vi "20200213_CHF_336.vi"() -> ()   [LabVIEW 2017]
uses:
  <vilib>/DAQmx/miscellaneous.llb/DAQmx Fill In Error Info.vi
  <vilib>/DAQmx/create/channels.llb/DAQmx Create Channel (AI-Voltage-Basic).vi
  <vilib>/DAQmx/create/channels.llb/DAQmx Create Channel (AO-Voltage-Basic).vi
  istr.lib/Lake Shore 336/Public/Data/Sensor Data (Single Reading).vi
  istr.lib/Lake Shore Cryotronics 218.lvlib
  istr.lib/Lake Shore 336/Lake Shore 336.lvlib
panel:
  in  "Tab Control":T1(tab)=enum."graphs"
  out "error out\n(file creation)":errorcluster
  out "error out\n(DAQ config)":errorcluster
  out "error out (LSI)":errorcluster
  out "error out (decoration)":errorcluster
  out "error out (DAQ AOU)":errorcluster
  out "error out (DAQ AIN)":errorcluster
  out "DAQ AIN task out":refnum<k21>="20200318_131117_AI"
  out "error out (end)":errorcluster
  in  "comments LSIU (not recorded)":string[](array[string])=["PtCo", "", "", "", "CERNOX", "CERNOX", "CERNOX", "CERNOX"]
  in  "LSI-U CH labels":string[](array[string])=["NC", "NC", "NC", "NC", "NC", "NC", "NC", "NC"]
  in  "DAQ-AIN labels":string[](array[string])=["P_4KRES", "LM_110", "DP_3He", "DP_4He", "FM_4He", "FM_3He", "LM_1700", "P_3He_IN", "P_3He_OUT", "P_bar_front", "Heater_V", "Heater_I", "LD_exponent", "LD_mantissa", "LD_full"]
  in  "DAQ AIN channels":tag[](array[tag])=["Dev1/ai1", "Dev1/ai2", "Dev1/ai3", "Dev1/ai4", "Dev1/ai5", "Dev1/ai6", "Dev1/ai7", "Dev1/ai16", "Dev1/ai17", "Dev1/ai18", "Dev1/ai19", "Dev1/ai23", "Dev1/ai21", "Dev1/ai22"]
  in  "V_min(in)":dbl[](array[numeric])=[0.0, 0.0, 0.0, 0.0, 0.0, 0.0, 0.0, 0.0, 0.0, 0.0, 0.0, 0.0, 0.0, 0.0]
  in  "V_max(in)":dbl[](array[numeric])=[5.0, 0.15, 5.0, 5.0, 5.0, 5.0, 10.0, 5.0, 5.0, 5.0, 10.0, 10.0, 10.0, 10.0]
  in  "comments DAQ (not recorded)":string[](array[string])=["", "", "pressure diff., range : 0-20kPa", "pressure diff., rrange : 0-1kPa", "", "", "The range of this is 0-10VDC", "absoulte pressure, 1-5V <-> 0-200kPa", "absoulte pressure, 1-5V <-> 0-200kPa", "baratron analog out ", "voltage over the heater via a voltage divider ", "current in A which flows through the heater", "leak detector readou exponent ", "leak detector readout mantissa"]
  in  "DAQ sample #":i32=5
  in  "LSI-D CH labels":string[](array[string])=["Helium", "Cu", "NC", "NC", "NC", "NC", "NC", "NC"]
  in  "comments LSID (not recorded)":string[](array[string])=["", "", "PtCo", "PtCo", "CERNOX", "CERNOX", "CERNOX", "CERNOX"]
  in  "VISA LSI218 UP":refnum<visa-resource-name>="GPIB0::8::INSTR"
  in  "VISA LSI336":refnum<visa-resource-name>="GPIB0::1::INSTR"
  in  "Rv/(Rv+Ro)":dbl=0.0907441 format="%_7f"
  in  "Ri (Ohm)":dbl=10.1 format="%_4f"
  out "DAQ AIN CONV":dbl[](array[numeric])=[-48461.36222166339, -0.034257721777445925, 46.07595449774182, 23.305171113781608, 0.6935562473065429, 0.15116757050047003, 0.036201034541511884, 100765.895313031, 101089.75178250414, 99597.26569585872, 0.010176692246159401, -5.8343379889446384e-05, -2.0, -0.004535554012344961, -4.535554012344961e-05]
  out "DAQ RAW":dbl[](array[numeric])=[0.04675189478348817, -0.00015003007966136236, 1.0071438225092348, 1.102328129093408, 0.014037402194859598, -0.0002649139326618283, 0.0025019891266333943, 3.0153836639221887, 3.0379056620474696, 3.940429396233107, -0.0017731538983390277, -0.00012886811862497516, 0.009407989382065898, -0.0011154395863216121, 0.0]
  out "LSI-D CH indic.":string[](array[string])=["Helium", "Cu", "NC", "NC", "NC", "NC", "NC", "NC"]
  out "LSI-D out":dbl[](array[numeric])=[0.0, 0.0, 1.213, 0.0, 0.0, 0.0, 4.0, 4.0]
  out "LSI-U CH indic,":string[](array[string])=["NC", "NC", "NC", "NC", "NC", "NC", "NC", "NC"]
  out "LSI-U out":dbl[](array[numeric])=[286.694, 286.481, 0.0, 0.0, 0.0, 0.0, 0.0, 0.0]
  out "DAQ AIN CH indic.":string[](array[string])=["P_4KRES", "LM_110", "DP_3He", "DP_4He", "FM_4He", "FM_3He", "LM_1700", "P_3He_IN", "P_3He_OUT", "P_bar_front", "Heater_V", "Heater_I", "LD_exponent", "LD_mantissa", "LD_full"]
  in  "log/linear 4":bool
  out "Graph LSI-D 1":cluster{dbl[], dbl[]}[](graph)=[{[3667349478.0127354, 3667349479.0140834, 3667349480.0134497, 3667349481.013572, 3667349482.014925, 3667349483.014216, 3667349484.015578, 3667349485.016135, 3667349486.016583, 3667349487.0163903, 3667349488.0179815, 3667349489.018835, 3667349490.018664, 3667349491.0187654, 3667349492.0187993, 3667349493.019667, 3667349494.019672, 3667349495.0196695, 3667349496.019436, 3667349497.021096, 3667349498.0206184], [0.0, 0.0, 0.0, 0.0, 0.0, 0.0, 0.0, 0.0, 0.0, 0.0, 0.0, 0.0, 0.0, 0.0, 0.0, 0.0, 0.0, 0.0, 0.0, 0.0, 0.0]}, {[3667349478.0127354, 3667349479.0140834, 3667349480.0134497, 3667349481.013572, 3667349482.014925, 3667349483.014216, 3667349484.015578, 3667349485.016135, 3667349486.016583, 3667349487.0163903, 3667349488.0179815, 3667349489.018835, 3667349490.018664, 3667349491.0187654, 3667349492.0187993, 3667349493.019667, 3667349494.019672, 3667349495.0196695, 3667349496.019436, 3667349497.021096, 3667349498.0206184], [0.0, 0.0, 0.0, 0.0, 0.0, 0.0, 0.0, 0.0, 0.0, 0.0, 0.0, 0.0, 0.0, 0.0, 0.0, 0.0, 0.0, 0.0, 0.0, 0.0, 0.0]}, {[3667349478.0127354, 3667349479.0140834, 3667349480.0134497, 3667349481.013572, 3667349482.014925, 3667349483.014216, 3667349484.015578, 3667349485.016135, 3667349486.016583, 3667349487.0163903, 3667349488.0179815, 3667349489.018835, 3667349490.018664, 3667349491.0187654, 3667349492.0187993, 3667349493.019667, 3667349494.019672, 3667349495.0196695, 3667349496.019436, 3667349497.021096, 3667349498.0206184], [1.213, 1.213, 1.213, 1.213, 1.213, 1.213, 1.213, 1.213, 1.213, 1.213, 1.213, 1.213, 1.213, 1.213, 1.213, 1.213, 1.213, 1.213, 1.213, 1.213, 1.213]}, {[3667349478.0127354, 3667349479.0140834, 3667349480.0134497, 3667349481.013572, 3667349482.014925, 3667349483.014216, 3667349484.015578, 3667349485.016135, 3667349486.016583, 3667349487.0163903, 3667349488.0179815, 3667349489.018835, 3667349490.018664, 3667349491.0187654, 3667349492.0187993, 3667349493.019667, 3667349494.019672, 3667349495.0196695, 3667349496.019436, 3667349497.021096, 3667349498.0206184], [0.0, 0.0, 0.0, 0.0, 0.0, 0.0, 0.0, 0.0, 0.0, 0.0, 0.0, 0.0, 0.0, 0.0, 0.0, 0.0, 0.0, 0.0, 0.0, 0.0, 0.0]}, {[3667349478.0127354, 3667349479.0140834, 3667349480.0134497, 3667349481.013572, 3667349482.014925, 3667349483.014216, 3667349484.015578, 3667349485.016135, 3667349486.016583, 3667349487.0163903, 3667349488.0179815, 3667349489.018835, 3667349490.018664, 3667349491.0187654, 3667349492.0187993, 3667349493.019667, 3667349494.019672, 3667349495.0196695, 3667349496.019436, 3667349497.021096, 3667349498.0206184], [0.0, 0.0, 0.0, 0.0, 0.0, 0.0, 0.0, 0.0, 0.0, 0.0, 0.0, 0.0, 0.0, 0.0, 0.0, 0.0, 0.0, 0.0, 0.0, 0.0, 0.0]}, {[3667349478.0127354, 3667349479.0140834, 3667349480.0134497, 3667349481.013572, 3667349482.014925, 3667349483.014216, 3667349484.015578, 3667349485.016135, 3667349486.016583, 3667349487.0163903, 3667349488.0179815, 3667349489.018835, 3667349490.018664, 3667349491.0187654, 3667349492.0187993, 3667349493.019667, 3667349494.019672, 3667349495.0196695, 3667349496.019436, 3667349497.021096, 3667349498.0206184], [0.0, 0.0, 0.0, 0.0, 0.0, 0.0, 0.0, 0.0, 0.0, 0.0, 0.0, 0.0, 0.0, 0.0, 0.0, 0.0, 0.0, 0.0, 0.0, 0.0, 0.0]}, {[3667349478.0127354, 3667349479.0140834, 3667349480.0134497, 3667349481.013572, 3667349482.014925, 3667349483.014216, 3667349484.015578, 3667349485.016135, 3667349486.016583, 3667349487.0163903, 3667349488.0179815, 3667349489.018835, 3667349490.018664, 3667349491.0187654, 3667349492.0187993, 3667349493.019667, 3667349494.019672, 3667349495.0196695, 3667349496.019436, 3667349497.021096, 3667349498.0206184], [4.0, 4.0, 4.0, 4.0, 4.0, 4.0, 4.0, 4.0, 4.0, 4.0, 4.0, 4.0, 4.0, 4.0, 4.0, 4.0, 4.0, 4.0, 4.0, 4.0, 4.0]}, {[3667349478.0127354, 3667349479.0140834, 3667349480.0134497, 3667349481.013572, 3667349482.014925, 3667349483.014216, 3667349484.015578, 3667349485.016135, 3667349486.016583, 3667349487.0163903, 3667349488.0179815, 3667349489.018835, 3667349490.018664, 3667349491.0187654, 3667349492.0187993, 3667349493.019667, 3667349494.019672, 3667349495.0196695, 3667349496.019436, 3667349497.021096, 3667349498.0206184], [4.0, 4.0, 4.0, 4.0, 4.0, 4.0, 4.0, 4.0, 4.0, 4.0, 4.0, 4.0, 4.0, 4.0, 4.0, 4.0, 4.0, 4.0, 4.0, 4.0, 4.0]}, {[3667349478.0127354, 3667349479.0140834, 3667349480.0134497, 3667349481.013572, 3667349482.014925, 3667349483.014216, 3667349484.015578, 3667349485.016135, 3667349486.016583, 3667349487.0163903, 3667349488.0179815, 3667349489.018835, 3667349490.018664, 3667349491.0187654, 3667349492.0187993, 3667349493.019667, 3667349494.019672, 3667349495.0196695, 3667349496.019436, 3667349497.021096, 3667349498.0206184], []}] caption="XY Graph"
  out "LSI-D out 1":dbl[](array[numeric])=[0.0, 0.0, 1.213, 0.0, 0.0, 0.0, 4.0, 4.0] format="%_3f"
  in  "log/linear 3":bool
  out "Graph S.1.3":cluster{dbl[], dbl[]}[](graph)=[{[3667349478.0127354, 3667349479.0140834, 3667349480.0134497, 3667349481.013572, 3667349482.014925, 3667349483.014216, 3667349484.015578, 3667349485.016135, 3667349486.016583, 3667349487.0163903, 3667349488.0179815, 3667349489.018835, 3667349490.018664, 3667349491.0187654, 3667349492.0187993, 3667349493.019667, 3667349494.019672, 3667349495.0196695, 3667349496.019436, 3667349497.021096, 3667349498.0206184], [-50521.2245456328, -51001.2563087499, -51385.9392869464, -50463.68651918715, -49646.64610974649, -49625.27485044931, -49894.88173933904, -50284.49655313725, -50743.15703962915, -50720.14180188283, -50039.54881966669, -49418.13787551146, -50679.04319398615, -49158.394647200206, -51098.24902658315, -50233.53425326837, -49625.27484957506, -50683.97503597823, -49748.570680075805, -49692.67657635927, -48461.36222166339]}, {[3667349478.0127354, 3667349479.0140834, 3667349480.0134497, 3667349481.013572, 3667349482.014925, 3667349483.014216, 3667349484.015578, 3667349485.016135, 3667349486.016583, 3667349487.0163903, 3667349488.0179815, 3667349489.018835, 3667349490.018664, 3667349491.0187654, 3667349492.0187993, 3667349493.019667, 3667349494.019672, 3667349495.0196695, 3667349496.019436, 3667349497.021096, 3667349498.0206184], [0.019681672163247236, -0.035573316743868315, -0.023732961916967353, -0.014523797115791916, -0.04609807649843742, 0.003894532544932317, -0.005314632339753402, -0.08425033110491678, -0.08161914105921124, -0.15660805460255026, -0.12898056031693128, -0.04215129156293204, -0.09609068567214586, -0.06714759614249097, 0.04073119171338225, -0.0026834424424830236, -0.13161175006152215, -0.07504116619060815, -0.05004486144342974, -0.043466886677967234, -0.034257721777445925]}, {[3667349478.0127354, 3667349479.0140834, 3667349480.0134497, 3667349481.013572, 3667349482.014925, 3667349483.014216, 3667349484.015578, 3667349485.016135, 3667349486.016583, 3667349487.0163903, 3667349488.0179815, 3667349489.018835, 3667349490.018664, 3667349491.0187654, 3667349492.0187993, 3667349493.019667, 3667349494.019672, 3667349495.0196695, 3667349496.019436, 3667349497.021096, 3667349498.0206184], [38.84260441471943, 39.006998855943834, 54.295670261381716, 29.965311373603143, 57.41916227904098, 16.649371673914672, 23.2251443857745, 16.978160296654554, 20.923623945936498, 25.855453443481835, 63.17296338630207, 33.74638070680503, 32.43122613515559, 37.363055655882384, 31.773648868628214, 29.965311397649465, 28.321368183241713, 23.882721679537866, 22.403172749733137, 59.22749982166353, 46.07595449774182]}, {[3667349478.0127354, 3667349479.0140834, 3667349480.0134497, 3667349481.013572, 3667349482.014925, 3667349483.014216, 3667349484.015578, 3667349485.016135, 3667349486.016583, 3667349487.0163903, 3667349488.0179815, 3667349489.018835, 3667349490.018664, 3667349491.0187654, 3667349492.0187993, 3667349493.019667, 3667349494.019672, 3667349495.0196695, 3667349496.019436, 3667349497.021096, 3667349498.0206184], [23.37092883661357, 22.721571321651922, 21.480394293207027, 24.02028635389264, 23.420247124279147, 23.08323879869223, 23.420247130213735, 22.713351606428176, 21.439295716348617, 23.214754246681622, 22.713351601179323, 23.206534532026367, 21.521492871998007, 22.828427616938708, 23.855892046718395, 22.129751813377673, 23.658618875732728, 22.302365835317307, 21.83384205492711, 21.54615201050991, 23.305171113781608]}, {[3667349478.0127354, 3667349479.0140834, 3667349480.0134497, 3667349481.013572, 3667349482.014925, 3667349483.014216, 3667349484.015578, 3667349485.016135, 3667349486.016583, 3667349487.0163903, 3667349488.0179815, 3667349489.018835, 3667349490.018664, 3667349491.0187654, 3667349492.0187993, 3667349493.019667, 3667349494.019672, 3667349495.0196695, 3667349496.019436, 3667349497.021096, 3667349498.0206184], [0.23982759672010165, 0.26941859522093714, 0.07872104719398296, 0.32531270582554006, -0.01662772910205959, -0.026491393526181937, 0.1806455987303783, 0.4897071440762254, -0.13170383494884252, 0.9565873491766973, 0.17078193234429023, 0.700132025147448, 0.6705410269020168, 0.627798472326523, 0.17406982087029635, 0.476555589056135, 0.48641925466059627, 0.0524179352505974, 0.21023659743522313, 0.06885738001278591, 0.6935562473065429]}, {[3667349478.0127354, 3667349479.0140834, 3667349480.0134497, 3667349481.013572, 3667349482.014925, 3667349483.014216, 3667349484.015578, 3667349485.016135, 3667349486.016583, 3667349487.0163903, 3667349488.0179815, 3667349489.018835, 3667349490.018664, 3667349491.0187654, 3667349492.0187993, 3667349493.019667, 3667349494.019672, 3667349495.0196695, 3667349496.019436, 3667349497.021096, 3667349498.0206184], [-0.0566270005152093, 0.19193739136287796, 0.1327553934585839, 0.15116757047502127, 0.14985241484089812, 0.028858107945263556, -0.040845134196314414, 0.09198557214999697, 0.09856134994531957, -0.08293011069980677, 0.11828868263099351, 0.009130775162069726, 0.07225823943248261, 0.09067041687947358, 0.06962792881441743, 0.10119166098595678, 0.11434321594263724, 0.047270285163107995, 0.024912641362354437, 0.18273130267201193, 0.15116757050047003]}, {[3667349478.0127354, 3667349479.0140834, 3667349480.0134497, 3667349481.013572, 3667349482.014925, 3667349483.014216, 3667349484.015578, 3667349485.016135, 3667349486.016583, 3667349487.0163903, 3667349488.0179815, 3667349489.018835, 3667349490.018664, 3667349491.0187654, 3667349492.0187993, 3667349493.019667, 3667349494.019672, 3667349495.0196695, 3667349496.019436, 3667349497.021096, 3667349498.0206184], [-0.920115595447706, -0.20123383292462396, -0.08218754169592701, 0.01712731949638921, 0.03488560589534542, 0.02304674833120446, 0.023046748329272143, 0.05132846367878108, 0.06514046419026112, 0.0217313197057645, 0.051328463673510655, 0.026335319880004177, 0.047382177823100224, 0.046724463511654324, 0.012523319345340012, -0.0045772527613157366, 0.011207890716825375, 0.015811890907051346, 0.04738217781528495, 0.055932463852581854, 0.036201034541511884]}, {[3667349478.0127354, 3667349479.0140834, 3667349480.0134497, 3667349481.013572, 3667349482.014925, 3667349483.014216, 3667349484.015578, 3667349485.016135, 3667349486.016583, 3667349487.0163903, 3667349488.0179815, 3667349489.018835, 3667349490.018664, 3667349491.0187654, 3667349492.0187993, 3667349493.019667, 3667349494.019672, 3667349495.0196695, 3667349496.019436, 3667349497.021096, 3667349498.0206184], [101084.81995907212, 100790.55443522778, 100880.97121607444, 100578.48598462425, 100890.83486492698, 100798.77414238652, 100728.08465890236, 100733.01648361162, 100821.78932327892, 100805.34990845669, 100811.92567437782, 100746.16801531675, 100894.1227478334, 100876.03939176453, 100568.62233567455, 100836.58479647475, 100622.87240454755, 100854.66815272612, 100912.20610427913, 100640.95576074878, 100765.895313031]}, {[3667349478.0127354, 3667349479.0140834, 3667349480.0134497, 3667349481.013572, 3667349482.014925, 3667349483.014216, 3667349484.015578, 3667349485.016135, 3667349486.016583, 3667349487.0163903, 3667349488.0179815, 3667349489.018835, 3667349490.018664, 3667349491.0187654, 3667349492.0187993, 3667349493.019667, 3667349494.019672, 3667349495.0196695, 3667349496.019436, 3667349497.021096, 3667349498.0206184], [101867.33609569666, 101987.34382303612, 100686.98611819187, 100535.74350397852, 101033.85777256651, 101078.24418841764, 101168.66097001858, 100936.86522534626, 101331.41117828828, 101622.3888165227, 101430.04766636596, 101250.85804619722, 101135.78214419658, 101701.29800932095, 101314.97176400454, 100908.91821834628, 100788.91049122188, 101416.8961349039, 101628.96458413133, 101282.0929351607, 101089.75178250414]}, {[3667349478.0127354, 3667349479.0140834, 3667349480.0134497, 3667349481.013572, 3667349482.014925, 3667349483.014216, 3667349484.015578, 3667349485.016135, 3667349486.016583, 3667349487.0163903, 3667349488.0179815, 3667349489.018835, 3667349490.018664, 3667349491.0187654, 3667349492.0187993, 3667349493.019667, 3667349494.019672, 3667349495.0196695, 3667349496.019436, 3667349497.021096, 3667349498.0206184], [101420.21419989626, 98144.87117860923, 98203.7358752945, 101313.85089177152, 101040.85716494694, 101526.68917410531, 101253.1219474301, 101465.83265061265, 100572.4245095208, 100965.15620313674, 101496.25635307128, 99254.47902652802, 101374.61625787482, 99209.8547871812, 101359.42150088456, 99746.67239306087, 99552.48733932934, 100316.46473552707, 100542.27772973066, 100889.51195743452, 99597.26569585872]}, {[3667349478.0127354, 3667349479.0140834, 3667349480.0134497, 3667349481.013572, 3667349482.014925, 3667349483.014216, 3667349484.015578, 3667349485.016135, 3667349486.016583, 3667349487.0163903, 3667349488.0179815, 3667349489.018835, 3667349490.018664, 3667349491.0187654, 3667349492.0187993, 3667349493.019667, 3667349494.019672, 3667349495.0196695, 3667349496.019436, 3667349497.021096, 3667349498.0206184], [0.018149505272345223, 0.0072774875169589, 0.00582788514456583, -0.00794333736102738, -0.010117740914873347, 0.018874306457283163, 0.006552686320306795, -0.00721853618344779, 0.019599107644447382, 0.00945189105599304, 0.015250300537917006, -0.002144927894012446, 0.009451891063447862, -0.020989758718289512, -0.012292144465621163, 0.0014790780319362934, 0.020323908801802685, -0.026788168204768564, 0.0007542768560017767, 0.0029286803972630835, 0.010176692246159401]}, {[3667349478.0127354, 3667349479.0140834, 3667349480.0134497, 3667349481.013572, 3667349482.014925, 3667349483.014216, 3667349484.015578, 3667349485.016135, 3667349486.016583, 3667349487.0163903, 3667349488.0179815, 3667349489.018835, 3667349490.018664, 3667349491.0187654, 3667349492.0187993, 3667349493.019667, 3667349494.019672, 3667349495.0196695, 3667349496.019436, 3667349497.021096, 3667349498.0206184], [2.648261071154278e-07, 2.6482610798491936e-07, 1.3288871881809514e-05, -6.247196779361987e-06, -3.2295288334838795e-05, 2.648261071154278e-07, 6.776848994462333e-06, -6.247196780231753e-06, -1.2759219666708891e-05, 6.776848996201591e-06, -3.229528833048914e-05, -1.927124255579533e-05, -1.9271242554925562e-05, 3.9336963428588106e-05, -6.247196783710818e-06, -1.9271242558404903e-05, -1.2759219669317917e-05, 2.6482610885468566e-07, -6.247196780231478e-06, -1.2759219666708891e-05, -5.8343379889446384e-05]}, {[3667349478.0127354, 3667349479.0140834, 3667349480.0134497, 3667349481.013572, 3667349482.014925, 3667349483.014216, 3667349484.015578, 3667349485.016135, 3667349486.016583, 3667349487.0163903, 3667349488.0179815, 3667349489.018835, 3667349490.018664, 3667349491.0187654, 3667349492.0187993, 3667349493.019667, 3667349494.019672, 3667349495.0196695, 3667349496.019436, 3667349497.021096, 3667349498.0206184], [-2.0, -2.0, -2.0, -2.0, -2.0, -2.0, -2.0, -2.0, -2.0, -2.0, -2.0, -2.0, -2.0, -2.0, -2.0, -2.0, -2.0, -2.0, -2.0, -2.0, -2.0]}, {[3667349478.0127354, 3667349479.0140834, 3667349480.0134497, 3667349481.013572, 3667349482.014925, 3667349483.014216, 3667349484.015578, 3667349485.016135, 3667349486.016583, 3667349487.0163903, 3667349488.0179815, 3667349489.018835, 3667349490.018664, 3667349491.0187654, 3667349492.0187993, 3667349493.019667, 3667349494.019672, 3667349495.0196695, 3667349496.019436, 3667349497.021096, 3667349498.0206184], [-0.07754184384077836, -0.0578104139341869, -0.04406418453851113, -0.033343441089875116, -0.024069669182046567, -0.01926835466596189, -0.014598583018555253, -0.01348046868200208, -0.012165040051646394, -0.008810697048266893, -0.009731497087684069, -0.009271097067931519, -0.010323439971000622, -0.00216778248702571, -0.0059825254999871375, -0.0075610398521598595, -0.006837554107855468, -0.0055878969121615305, -0.00696909697009179, -0.005456354050443748, -0.004535554012344961]}, {[3667349478.0127354, 3667349479.0140834, 3667349480.0134497, 3667349481.013572, 3667349482.014925, 3667349483.014216, 3667349484.015578, 3667349485.016135, 3667349486.016583, 3667349487.0163903, 3667349488.0179815, 3667349489.018835, 3667349490.018664, 3667349491.0187654, 3667349492.0187993, 3667349493.019667, 3667349494.019672, 3667349495.0196695, 3667349496.019436, 3667349497.021096, 3667349498.0206184], [-0.0007754184384077836, -0.000578104139341869, -0.00044064184538511133, -0.0003334344108987512, -0.00024069669182046568, -0.0001926835466596189, -0.00014598583018555252, -0.0001348046868200208, -0.00012165040051646394, -8.810697048266893e-05, -9.731497087684068e-05, -9.271097067931519e-05, -0.00010323439971000622, -2.1677824870257103e-05, -5.9825254999871375e-05, -7.561039852159859e-05, -6.837554107855468e-05, -5.58789691216153e-05, -6.96909697009179e-05, -5.4563540504437485e-05, -4.535554012344961e-05]}] caption="XY Graph"
  out "OUT S.1.3":dbl[](array[numeric])=[101479.36590743523, 30.884846138935902, 42.788068085590766, 19.787132912531703, 115.97017410165145, 0.14459179297742142, 0.47884275917250574, 101362.64606746232, 102150.09402793349, 100980.291856696, 0.03192072773109346, -3.805377120271886e-05, -2.0, 0.003225474858579311, 3.225474858579311e-05] format="%_4e"
  in  "log/linear 2":bool
  out "OUT S.1 1":dbl[](array[numeric])=[-48461.36222166339, -0.034257721777445925, 46.07595449774182, 23.305171113781608, 0.6935562473065429, 0.15116757050047003, 0.036201034541511884, 100765.895313031, 101089.75178250414, 99597.26569585872, 0.010176692246159401, -5.8343379889446384e-05, -2.0, -0.004535554012344961, -4.535554012344961e-05] format="%_4e"
  out "Graph S.1.1":cluster{dbl[], dbl[]}[](graph)=[{[3667349478.0127354, 3667349479.0140834, 3667349480.0134497, 3667349481.013572, 3667349482.014925, 3667349483.014216, 3667349484.015578, 3667349485.016135, 3667349486.016583, 3667349487.0163903, 3667349488.0179815, 3667349489.018835, 3667349490.018664, 3667349491.0187654, 3667349492.0187993, 3667349493.019667, 3667349494.019672, 3667349495.0196695, 3667349496.019436, 3667349497.021096, 3667349498.0206184], [-50521.2245456328, -51001.2563087499, -51385.9392869464, -50463.68651918715, -49646.64610974649, -49625.27485044931, -49894.88173933904, -50284.49655313725, -50743.15703962915, -50720.14180188283, -50039.54881966669, -49418.13787551146, -50679.04319398615, -49158.394647200206, -51098.24902658315, -50233.53425326837, -49625.27484957506, -50683.97503597823, -49748.570680075805, -49692.67657635927, -48461.36222166339]}, {[3667349478.0127354, 3667349479.0140834, 3667349480.0134497, 3667349481.013572, 3667349482.014925, 3667349483.014216, 3667349484.015578, 3667349485.016135, 3667349486.016583, 3667349487.0163903, 3667349488.0179815, 3667349489.018835, 3667349490.018664, 3667349491.0187654, 3667349492.0187993, 3667349493.019667, 3667349494.019672, 3667349495.0196695, 3667349496.019436, 3667349497.021096, 3667349498.0206184], [0.019681672163247236, -0.035573316743868315, -0.023732961916967353, -0.014523797115791916, -0.04609807649843742, 0.003894532544932317, -0.005314632339753402, -0.08425033110491678, -0.08161914105921124, -0.15660805460255026, -0.12898056031693128, -0.04215129156293204, -0.09609068567214586, -0.06714759614249097, 0.04073119171338225, -0.0026834424424830236, -0.13161175006152215, -0.07504116619060815, -0.05004486144342974, -0.043466886677967234, -0.034257721777445925]}, {[3667349478.0127354, 3667349479.0140834, 3667349480.0134497, 3667349481.013572, 3667349482.014925, 3667349483.014216, 3667349484.015578, 3667349485.016135, 3667349486.016583, 3667349487.0163903, 3667349488.0179815, 3667349489.018835, 3667349490.018664, 3667349491.0187654, 3667349492.0187993, 3667349493.019667, 3667349494.019672, 3667349495.0196695, 3667349496.019436, 3667349497.021096, 3667349498.0206184], [38.84260441471943, 39.006998855943834, 54.295670261381716, 29.965311373603143, 57.41916227904098, 16.649371673914672, 23.2251443857745, 16.978160296654554, 20.923623945936498, 25.855453443481835, 63.17296338630207, 33.74638070680503, 32.43122613515559, 37.363055655882384, 31.773648868628214, 29.965311397649465, 28.321368183241713, 23.882721679537866, 22.403172749733137, 59.22749982166353, 46.07595449774182]}, {[3667349478.0127354, 3667349479.0140834, 3667349480.0134497, 3667349481.013572, 3667349482.014925, 3667349483.014216, 3667349484.015578, 3667349485.016135, 3667349486.016583, 3667349487.0163903, 3667349488.0179815, 3667349489.018835, 3667349490.018664, 3667349491.0187654, 3667349492.0187993, 3667349493.019667, 3667349494.019672, 3667349495.0196695, 3667349496.019436, 3667349497.021096, 3667349498.0206184], [23.37092883661357, 22.721571321651922, 21.480394293207027, 24.02028635389264, 23.420247124279147, 23.08323879869223, 23.420247130213735, 22.713351606428176, 21.439295716348617, 23.214754246681622, 22.713351601179323, 23.206534532026367, 21.521492871998007, 22.828427616938708, 23.855892046718395, 22.129751813377673, 23.658618875732728, 22.302365835317307, 21.83384205492711, 21.54615201050991, 23.305171113781608]}, {[3667349478.0127354, 3667349479.0140834, 3667349480.0134497, 3667349481.013572, 3667349482.014925, 3667349483.014216, 3667349484.015578, 3667349485.016135, 3667349486.016583, 3667349487.0163903, 3667349488.0179815, 3667349489.018835, 3667349490.018664, 3667349491.0187654, 3667349492.0187993, 3667349493.019667, 3667349494.019672, 3667349495.0196695, 3667349496.019436, 3667349497.021096, 3667349498.0206184], [0.23982759672010165, 0.26941859522093714, 0.07872104719398296, 0.32531270582554006, -0.01662772910205959, -0.026491393526181937, 0.1806455987303783, 0.4897071440762254, -0.13170383494884252, 0.9565873491766973, 0.17078193234429023, 0.700132025147448, 0.6705410269020168, 0.627798472326523, 0.17406982087029635, 0.476555589056135, 0.48641925466059627, 0.0524179352505974, 0.21023659743522313, 0.06885738001278591, 0.6935562473065429]}, {[3667349478.0127354, 3667349479.0140834, 3667349480.0134497, 3667349481.013572, 3667349482.014925, 3667349483.014216, 3667349484.015578, 3667349485.016135, 3667349486.016583, 3667349487.0163903, 3667349488.0179815, 3667349489.018835, 3667349490.018664, 3667349491.0187654, 3667349492.0187993, 3667349493.019667, 3667349494.019672, 3667349495.0196695, 3667349496.019436, 3667349497.021096, 3667349498.0206184], [-0.0566270005152093, 0.19193739136287796, 0.1327553934585839, 0.15116757047502127, 0.14985241484089812, 0.028858107945263556, -0.040845134196314414, 0.09198557214999697, 0.09856134994531957, -0.08293011069980677, 0.11828868263099351, 0.009130775162069726, 0.07225823943248261, 0.09067041687947358, 0.06962792881441743, 0.10119166098595678, 0.11434321594263724, 0.047270285163107995, 0.024912641362354437, 0.18273130267201193, 0.15116757050047003]}, {[3667349478.0127354, 3667349479.0140834, 3667349480.0134497, 3667349481.013572, 3667349482.014925, 3667349483.014216, 3667349484.015578, 3667349485.016135, 3667349486.016583, 3667349487.0163903, 3667349488.0179815, 3667349489.018835, 3667349490.018664, 3667349491.0187654, 3667349492.0187993, 3667349493.019667, 3667349494.019672, 3667349495.0196695, 3667349496.019436, 3667349497.021096, 3667349498.0206184], [-0.920115595447706, -0.20123383292462396, -0.08218754169592701, 0.01712731949638921, 0.03488560589534542, 0.02304674833120446, 0.023046748329272143, 0.05132846367878108, 0.06514046419026112, 0.0217313197057645, 0.051328463673510655, 0.026335319880004177, 0.047382177823100224, 0.046724463511654324, 0.012523319345340012, -0.0045772527613157366, 0.011207890716825375, 0.015811890907051346, 0.04738217781528495, 0.055932463852581854, 0.036201034541511884]}, {[3667349478.0127354, 3667349479.0140834, 3667349480.0134497, 3667349481.013572, 3667349482.014925, 3667349483.014216, 3667349484.015578, 3667349485.016135, 3667349486.016583, 3667349487.0163903, 3667349488.0179815, 3667349489.018835, 3667349490.018664, 3667349491.0187654, 3667349492.0187993, 3667349493.019667, 3667349494.019672, 3667349495.0196695, 3667349496.019436, 3667349497.021096, 3667349498.0206184], [101084.81995907212, 100790.55443522778, 100880.97121607444, 100578.48598462425, 100890.83486492698, 100798.77414238652, 100728.08465890236, 100733.01648361162, 100821.78932327892, 100805.34990845669, 100811.92567437782, 100746.16801531675, 100894.1227478334, 100876.03939176453, 100568.62233567455, 100836.58479647475, 100622.87240454755, 100854.66815272612, 100912.20610427913, 100640.95576074878, 100765.895313031]}, {[3667349478.0127354, 3667349479.0140834, 3667349480.0134497, 3667349481.013572, 3667349482.014925, 3667349483.014216, 3667349484.015578, 3667349485.016135, 3667349486.016583, 3667349487.0163903, 3667349488.0179815, 3667349489.018835, 3667349490.018664, 3667349491.0187654, 3667349492.0187993, 3667349493.019667, 3667349494.019672, 3667349495.0196695, 3667349496.019436, 3667349497.021096, 3667349498.0206184], [101867.33609569666, 101987.34382303612, 100686.98611819187, 100535.74350397852, 101033.85777256651, 101078.24418841764, 101168.66097001858, 100936.86522534626, 101331.41117828828, 101622.3888165227, 101430.04766636596, 101250.85804619722, 101135.78214419658, 101701.29800932095, 101314.97176400454, 100908.91821834628, 100788.91049122188, 101416.8961349039, 101628.96458413133, 101282.0929351607, 101089.75178250414]}, {[3667349478.0127354, 3667349479.0140834, 3667349480.0134497, 3667349481.013572, 3667349482.014925, 3667349483.014216, 3667349484.015578, 3667349485.016135, 3667349486.016583, 3667349487.0163903, 3667349488.0179815, 3667349489.018835, 3667349490.018664, 3667349491.0187654, 3667349492.0187993, 3667349493.019667, 3667349494.019672, 3667349495.0196695, 3667349496.019436, 3667349497.021096, 3667349498.0206184], [101420.21419989626, 98144.87117860923, 98203.7358752945, 101313.85089177152, 101040.85716494694, 101526.68917410531, 101253.1219474301, 101465.83265061265, 100572.4245095208, 100965.15620313674, 101496.25635307128, 99254.47902652802, 101374.61625787482, 99209.8547871812, 101359.42150088456, 99746.67239306087, 99552.48733932934, 100316.46473552707, 100542.27772973066, 100889.51195743452, 99597.26569585872]}, {[3667349478.0127354, 3667349479.0140834, 3667349480.0134497, 3667349481.013572, 3667349482.014925, 3667349483.014216, 3667349484.015578, 3667349485.016135, 3667349486.016583, 3667349487.0163903, 3667349488.0179815, 3667349489.018835, 3667349490.018664, 3667349491.0187654, 3667349492.0187993, 3667349493.019667, 3667349494.019672, 3667349495.0196695, 3667349496.019436, 3667349497.021096, 3667349498.0206184], [0.018149505272345223, 0.0072774875169589, 0.00582788514456583, -0.00794333736102738, -0.010117740914873347, 0.018874306457283163, 0.006552686320306795, -0.00721853618344779, 0.019599107644447382, 0.00945189105599304, 0.015250300537917006, -0.002144927894012446, 0.009451891063447862, -0.020989758718289512, -0.012292144465621163, 0.0014790780319362934, 0.020323908801802685, -0.026788168204768564, 0.0007542768560017767, 0.0029286803972630835, 0.010176692246159401]}, {[3667349478.0127354, 3667349479.0140834, 3667349480.0134497, 3667349481.013572, 3667349482.014925, 3667349483.014216, 3667349484.015578, 3667349485.016135, 3667349486.016583, 3667349487.0163903, 3667349488.0179815, 3667349489.018835, 3667349490.018664, 3667349491.0187654, 3667349492.0187993, 3667349493.019667, 3667349494.019672, 3667349495.0196695, 3667349496.019436, 3667349497.021096, 3667349498.0206184], [2.648261071154278e-07, 2.6482610798491936e-07, 1.3288871881809514e-05, -6.247196779361987e-06, -3.2295288334838795e-05, 2.648261071154278e-07, 6.776848994462333e-06, -6.247196780231753e-06, -1.2759219666708891e-05, 6.776848996201591e-06, -3.229528833048914e-05, -1.927124255579533e-05, -1.9271242554925562e-05, 3.9336963428588106e-05, -6.247196783710818e-06, -1.9271242558404903e-05, -1.2759219669317917e-05, 2.6482610885468566e-07, -6.247196780231478e-06, -1.2759219666708891e-05, -5.8343379889446384e-05]}, {[3667349478.0127354, 3667349479.0140834, 3667349480.0134497, 3667349481.013572, 3667349482.014925, 3667349483.014216, 3667349484.015578, 3667349485.016135, 3667349486.016583, 3667349487.0163903, 3667349488.0179815, 3667349489.018835, 3667349490.018664, 3667349491.0187654, 3667349492.0187993, 3667349493.019667, 3667349494.019672, 3667349495.0196695, 3667349496.019436, 3667349497.021096, 3667349498.0206184], [-2.0, -2.0, -2.0, -2.0, -2.0, -2.0, -2.0, -2.0, -2.0, -2.0, -2.0, -2.0, -2.0, -2.0, -2.0, -2.0, -2.0, -2.0, -2.0, -2.0, -2.0]}, {[3667349478.0127354, 3667349479.0140834, 3667349480.0134497, 3667349481.013572, 3667349482.014925, 3667349483.014216, 3667349484.015578, 3667349485.016135, 3667349486.016583, 3667349487.0163903, 3667349488.0179815, 3667349489.018835, 3667349490.018664, 3667349491.0187654, 3667349492.0187993, 3667349493.019667, 3667349494.019672, 3667349495.0196695, 3667349496.019436, 3667349497.021096, 3667349498.0206184], [-0.07754184384077836, -0.0578104139341869, -0.04406418453851113, -0.033343441089875116, -0.024069669182046567, -0.01926835466596189, -0.014598583018555253, -0.01348046868200208, -0.012165040051646394, -0.008810697048266893, -0.009731497087684069, -0.009271097067931519, -0.010323439971000622, -0.00216778248702571, -0.0059825254999871375, -0.0075610398521598595, -0.006837554107855468, -0.0055878969121615305, -0.00696909697009179, -0.005456354050443748, -0.004535554012344961]}, {[3667349478.0127354, 3667349479.0140834, 3667349480.0134497, 3667349481.013572, 3667349482.014925, 3667349483.014216, 3667349484.015578, 3667349485.016135, 3667349486.016583, 3667349487.0163903, 3667349488.0179815, 3667349489.018835, 3667349490.018664, 3667349491.0187654, 3667349492.0187993, 3667349493.019667, 3667349494.019672, 3667349495.0196695, 3667349496.019436, 3667349497.021096, 3667349498.0206184], [-0.0007754184384077836, -0.000578104139341869, -0.00044064184538511133, -0.0003334344108987512, -0.00024069669182046568, -0.0001926835466596189, -0.00014598583018555252, -0.0001348046868200208, -0.00012165040051646394, -8.810697048266893e-05, -9.731497087684068e-05, -9.271097067931519e-05, -0.00010323439971000622, -2.1677824870257103e-05, -5.9825254999871375e-05, -7.561039852159859e-05, -6.837554107855468e-05, -5.58789691216153e-05, -6.96909697009179e-05, -5.4563540504437485e-05, -4.535554012344961e-05]}] caption="XY Graph"
  out "Graph S.1.2":cluster{dbl[], dbl[]}[](graph)=[{[3667349478.0127354, 3667349479.0140834, 3667349480.0134497, 3667349481.013572, 3667349482.014925, 3667349483.014216, 3667349484.015578, 3667349485.016135, 3667349486.016583, 3667349487.0163903, 3667349488.0179815, 3667349489.018835, 3667349490.018664, 3667349491.0187654, 3667349492.0187993, 3667349493.019667, 3667349494.019672, 3667349495.0196695, 3667349496.019436, 3667349497.021096, 3667349498.0206184], [-50521.2245456328, -51001.2563087499, -51385.9392869464, -50463.68651918715, -49646.64610974649, -49625.27485044931, -49894.88173933904, -50284.49655313725, -50743.15703962915, -50720.14180188283, -50039.54881966669, -49418.13787551146, -50679.04319398615, -49158.394647200206, -51098.24902658315, -50233.53425326837, -49625.27484957506, -50683.97503597823, -49748.570680075805, -49692.67657635927, -48461.36222166339]}, {[3667349478.0127354, 3667349479.0140834, 3667349480.0134497, 3667349481.013572, 3667349482.014925, 3667349483.014216, 3667349484.015578, 3667349485.016135, 3667349486.016583, 3667349487.0163903, 3667349488.0179815, 3667349489.018835, 3667349490.018664, 3667349491.0187654, 3667349492.0187993, 3667349493.019667, 3667349494.019672, 3667349495.0196695, 3667349496.019436, 3667349497.021096, 3667349498.0206184], [0.019681672163247236, -0.035573316743868315, -0.023732961916967353, -0.014523797115791916, -0.04609807649843742, 0.003894532544932317, -0.005314632339753402, -0.08425033110491678, -0.08161914105921124, -0.15660805460255026, -0.12898056031693128, -0.04215129156293204, -0.09609068567214586, -0.06714759614249097, 0.04073119171338225, -0.0026834424424830236, -0.13161175006152215, -0.07504116619060815, -0.05004486144342974, -0.043466886677967234, -0.034257721777445925]}, {[3667349478.0127354, 3667349479.0140834, 3667349480.0134497, 3667349481.013572, 3667349482.014925, 3667349483.014216, 3667349484.015578, 3667349485.016135, 3667349486.016583, 3667349487.0163903, 3667349488.0179815, 3667349489.018835, 3667349490.018664, 3667349491.0187654, 3667349492.0187993, 3667349493.019667, 3667349494.019672, 3667349495.0196695, 3667349496.019436, 3667349497.021096, 3667349498.0206184], [38.84260441471943, 39.006998855943834, 54.295670261381716, 29.965311373603143, 57.41916227904098, 16.649371673914672, 23.2251443857745, 16.978160296654554, 20.923623945936498, 25.855453443481835, 63.17296338630207, 33.74638070680503, 32.43122613515559, 37.363055655882384, 31.773648868628214, 29.965311397649465, 28.321368183241713, 23.882721679537866, 22.403172749733137, 59.22749982166353, 46.07595449774182]}, {[3667349478.0127354, 3667349479.0140834, 3667349480.0134497, 3667349481.013572, 3667349482.014925, 3667349483.014216, 3667349484.015578, 3667349485.016135, 3667349486.016583, 3667349487.0163903, 3667349488.0179815, 3667349489.018835, 3667349490.018664, 3667349491.0187654, 3667349492.0187993, 3667349493.019667, 3667349494.019672, 3667349495.0196695, 3667349496.019436, 3667349497.021096, 3667349498.0206184], [23.37092883661357, 22.721571321651922, 21.480394293207027, 24.02028635389264, 23.420247124279147, 23.08323879869223, 23.420247130213735, 22.713351606428176, 21.439295716348617, 23.214754246681622, 22.713351601179323, 23.206534532026367, 21.521492871998007, 22.828427616938708, 23.855892046718395, 22.129751813377673, 23.658618875732728, 22.302365835317307, 21.83384205492711, 21.54615201050991, 23.305171113781608]}, {[3667349478.0127354, 3667349479.0140834, 3667349480.0134497, 3667349481.013572, 3667349482.014925, 3667349483.014216, 3667349484.015578, 3667349485.016135, 3667349486.016583, 3667349487.0163903, 3667349488.0179815, 3667349489.018835, 3667349490.018664, 3667349491.0187654, 3667349492.0187993, 3667349493.019667, 3667349494.019672, 3667349495.0196695, 3667349496.019436, 3667349497.021096, 3667349498.0206184], [0.23982759672010165, 0.26941859522093714, 0.07872104719398296, 0.32531270582554006, -0.01662772910205959, -0.026491393526181937, 0.1806455987303783, 0.4897071440762254, -0.13170383494884252, 0.9565873491766973, 0.17078193234429023, 0.700132025147448, 0.6705410269020168, 0.627798472326523, 0.17406982087029635, 0.476555589056135, 0.48641925466059627, 0.0524179352505974, 0.21023659743522313, 0.06885738001278591, 0.6935562473065429]}, {[3667349478.0127354, 3667349479.0140834, 3667349480.0134497, 3667349481.013572, 3667349482.014925, 3667349483.014216, 3667349484.015578, 3667349485.016135, 3667349486.016583, 3667349487.0163903, 3667349488.0179815, 3667349489.018835, 3667349490.018664, 3667349491.0187654, 3667349492.0187993, 3667349493.019667, 3667349494.019672, 3667349495.0196695, 3667349496.019436, 3667349497.021096, 3667349498.0206184], [-0.0566270005152093, 0.19193739136287796, 0.1327553934585839, 0.15116757047502127, 0.14985241484089812, 0.028858107945263556, -0.040845134196314414, 0.09198557214999697, 0.09856134994531957, -0.08293011069980677, 0.11828868263099351, 0.009130775162069726, 0.07225823943248261, 0.09067041687947358, 0.06962792881441743, 0.10119166098595678, 0.11434321594263724, 0.047270285163107995, 0.024912641362354437, 0.18273130267201193, 0.15116757050047003]}, {[3667349478.0127354, 3667349479.0140834, 3667349480.0134497, 3667349481.013572, 3667349482.014925, 3667349483.014216, 3667349484.015578, 3667349485.016135, 3667349486.016583, 3667349487.0163903, 3667349488.0179815, 3667349489.018835, 3667349490.018664, 3667349491.0187654, 3667349492.0187993, 3667349493.019667, 3667349494.019672, 3667349495.0196695, 3667349496.019436, 3667349497.021096, 3667349498.0206184], [-0.920115595447706, -0.20123383292462396, -0.08218754169592701, 0.01712731949638921, 0.03488560589534542, 0.02304674833120446, 0.023046748329272143, 0.05132846367878108, 0.06514046419026112, 0.0217313197057645, 0.051328463673510655, 0.026335319880004177, 0.047382177823100224, 0.046724463511654324, 0.012523319345340012, -0.0045772527613157366, 0.011207890716825375, 0.015811890907051346, 0.04738217781528495, 0.055932463852581854, 0.036201034541511884]}, {[3667349478.0127354, 3667349479.0140834, 3667349480.0134497, 3667349481.013572, 3667349482.014925, 3667349483.014216, 3667349484.015578, 3667349485.016135, 3667349486.016583, 3667349487.0163903, 3667349488.0179815, 3667349489.018835, 3667349490.018664, 3667349491.0187654, 3667349492.0187993, 3667349493.019667, 3667349494.019672, 3667349495.0196695, 3667349496.019436, 3667349497.021096, 3667349498.0206184], [101084.81995907212, 100790.55443522778, 100880.97121607444, 100578.48598462425, 100890.83486492698, 100798.77414238652, 100728.08465890236, 100733.01648361162, 100821.78932327892, 100805.34990845669, 100811.92567437782, 100746.16801531675, 100894.1227478334, 100876.03939176453, 100568.62233567455, 100836.58479647475, 100622.87240454755, 100854.66815272612, 100912.20610427913, 100640.95576074878, 100765.895313031]}, {[3667349478.0127354, 3667349479.0140834, 3667349480.0134497, 3667349481.013572, 3667349482.014925, 3667349483.014216, 3667349484.015578, 3667349485.016135, 3667349486.016583, 3667349487.0163903, 3667349488.0179815, 3667349489.018835, 3667349490.018664, 3667349491.0187654, 3667349492.0187993, 3667349493.019667, 3667349494.019672, 3667349495.0196695, 3667349496.019436, 3667349497.021096, 3667349498.0206184], [101867.33609569666, 101987.34382303612, 100686.98611819187, 100535.74350397852, 101033.85777256651, 101078.24418841764, 101168.66097001858, 100936.86522534626, 101331.41117828828, 101622.3888165227, 101430.04766636596, 101250.85804619722, 101135.78214419658, 101701.29800932095, 101314.97176400454, 100908.91821834628, 100788.91049122188, 101416.8961349039, 101628.96458413133, 101282.0929351607, 101089.75178250414]}, {[3667349478.0127354, 3667349479.0140834, 3667349480.0134497, 3667349481.013572, 3667349482.014925, 3667349483.014216, 3667349484.015578, 3667349485.016135, 3667349486.016583, 3667349487.0163903, 3667349488.0179815, 3667349489.018835, 3667349490.018664, 3667349491.0187654, 3667349492.0187993, 3667349493.019667, 3667349494.019672, 3667349495.0196695, 3667349496.019436, 3667349497.021096, 3667349498.0206184], [101420.21419989626, 98144.87117860923, 98203.7358752945, 101313.85089177152, 101040.85716494694, 101526.68917410531, 101253.1219474301, 101465.83265061265, 100572.4245095208, 100965.15620313674, 101496.25635307128, 99254.47902652802, 101374.61625787482, 99209.8547871812, 101359.42150088456, 99746.67239306087, 99552.48733932934, 100316.46473552707, 100542.27772973066, 100889.51195743452, 99597.26569585872]}, {[3667349478.0127354, 3667349479.0140834, 3667349480.0134497, 3667349481.013572, 3667349482.014925, 3667349483.014216, 3667349484.015578, 3667349485.016135, 3667349486.016583, 3667349487.0163903, 3667349488.0179815, 3667349489.018835, 3667349490.018664, 3667349491.0187654, 3667349492.0187993, 3667349493.019667, 3667349494.019672, 3667349495.0196695, 3667349496.019436, 3667349497.021096, 3667349498.0206184], [0.018149505272345223, 0.0072774875169589, 0.00582788514456583, -0.00794333736102738, -0.010117740914873347, 0.018874306457283163, 0.006552686320306795, -0.00721853618344779, 0.019599107644447382, 0.00945189105599304, 0.015250300537917006, -0.002144927894012446, 0.009451891063447862, -0.020989758718289512, -0.012292144465621163, 0.0014790780319362934, 0.020323908801802685, -0.026788168204768564, 0.0007542768560017767, 0.0029286803972630835, 0.010176692246159401]}, {[3667349478.0127354, 3667349479.0140834, 3667349480.0134497, 3667349481.013572, 3667349482.014925, 3667349483.014216, 3667349484.015578, 3667349485.016135, 3667349486.016583, 3667349487.0163903, 3667349488.0179815, 3667349489.018835, 3667349490.018664, 3667349491.0187654, 3667349492.0187993, 3667349493.019667, 3667349494.019672, 3667349495.0196695, 3667349496.019436, 3667349497.021096, 3667349498.0206184], [2.648261071154278e-07, 2.6482610798491936e-07, 1.3288871881809514e-05, -6.247196779361987e-06, -3.2295288334838795e-05, 2.648261071154278e-07, 6.776848994462333e-06, -6.247196780231753e-06, -1.2759219666708891e-05, 6.776848996201591e-06, -3.229528833048914e-05, -1.927124255579533e-05, -1.9271242554925562e-05, 3.9336963428588106e-05, -6.247196783710818e-06, -1.9271242558404903e-05, -1.2759219669317917e-05, 2.6482610885468566e-07, -6.247196780231478e-06, -1.2759219666708891e-05, -5.8343379889446384e-05]}, {[3667349478.0127354, 3667349479.0140834, 3667349480.0134497, 3667349481.013572, 3667349482.014925, 3667349483.014216, 3667349484.015578, 3667349485.016135, 3667349486.016583, 3667349487.0163903, 3667349488.0179815, 3667349489.018835, 3667349490.018664, 3667349491.0187654, 3667349492.0187993, 3667349493.019667, 3667349494.019672, 3667349495.0196695, 3667349496.019436, 3667349497.021096, 3667349498.0206184], [-2.0, -2.0, -2.0, -2.0, -2.0, -2.0, -2.0, -2.0, -2.0, -2.0, -2.0, -2.0, -2.0, -2.0, -2.0, -2.0, -2.0, -2.0, -2.0, -2.0, -2.0]}, {[3667349478.0127354, 3667349479.0140834, 3667349480.0134497, 3667349481.013572, 3667349482.014925, 3667349483.014216, 3667349484.015578, 3667349485.016135, 3667349486.016583, 3667349487.0163903, 3667349488.0179815, 3667349489.018835, 3667349490.018664, 3667349491.0187654, 3667349492.0187993, 3667349493.019667, 3667349494.019672, 3667349495.0196695, 3667349496.019436, 3667349497.021096, 3667349498.0206184], [-0.07754184384077836, -0.0578104139341869, -0.04406418453851113, -0.033343441089875116, -0.024069669182046567, -0.01926835466596189, -0.014598583018555253, -0.01348046868200208, -0.012165040051646394, -0.008810697048266893, -0.009731497087684069, -0.009271097067931519, -0.010323439971000622, -0.00216778248702571, -0.0059825254999871375, -0.0075610398521598595, -0.006837554107855468, -0.0055878969121615305, -0.00696909697009179, -0.005456354050443748, -0.004535554012344961]}, {[3667349478.0127354, 3667349479.0140834, 3667349480.0134497, 3667349481.013572, 3667349482.014925, 3667349483.014216, 3667349484.015578, 3667349485.016135, 3667349486.016583, 3667349487.0163903, 3667349488.0179815, 3667349489.018835, 3667349490.018664, 3667349491.0187654, 3667349492.0187993, 3667349493.019667, 3667349494.019672, 3667349495.0196695, 3667349496.019436, 3667349497.021096, 3667349498.0206184], [-0.0007754184384077836, -0.000578104139341869, -0.00044064184538511133, -0.0003334344108987512, -0.00024069669182046568, -0.0001926835466596189, -0.00014598583018555252, -0.0001348046868200208, -0.00012165040051646394, -8.810697048266893e-05, -9.731497087684068e-05, -9.271097067931519e-05, -0.00010323439971000622, -2.1677824870257103e-05, -5.9825254999871375e-05, -7.561039852159859e-05, -6.837554107855468e-05, -5.58789691216153e-05, -6.96909697009179e-05, -5.4563540504437485e-05, -4.535554012344961e-05]}] caption="XY Graph"
  out "OUT S.1.2":dbl[](array[numeric])=[-48461.36222166339, -0.034257721777445925, 46.07595449774182, 23.305171113781608, 0.6935562473065429, 0.15116757050047003, 0.036201034541511884, 100765.895313031, 101089.75178250414, 99597.26569585872, 0.010176692246159401, -5.8343379889446384e-05, -2.0, -0.004535554012344961, -4.535554012344961e-05] format="%_4e"
  in  "log/linear 1":bool
  in  "Tab Control 2":enum32{"config", "control"}(tab)=enum."control"
  in  "DAQ AOUT ch":tag="Dev1/ao1"
  in  "DAQ-AOUT labels":string="Hetaer_CTRL"
  out "DAQ AOUT task out":refnum<k21>="20200318_131117_AO"
  in  "V_lim_min":dbl min=0.0 max=110.0
  in  "V_lim_max":dbl=10.0 min=0.0 max=110.0
  in  "Record Boling curve":bool
  in  "DAQ-O \nAUTO CTL":bool
  in  "DAQ OUT MIN (V)":dbl format="%.5f"
  in  "DAQ OUT MAX (V)":dbl=40.0 format="%.5f"
  in  "dV/cycle (V)":dbl=-0.02 format="%_4f"
  in  "dt (ms) (>50)":u32=200 min=30
  in  "DAQ OUT SET V":dbl=2.706168622523819e-16 min=0.0 max=110.0 format="%_5f"
  out "Vctrl":dbl=2.460153293203472e-17 format="%_5f"
  in  "DAQ OUT ON?":bool
  out "cycle # CTRL":i32=1
  out "Graph BC":cluster{dbl[], dbl[]}(graph)={[-0.19700000000000273, -0.19700000000000273, -0.19700000000000273, -0.19700000000000273, -0.19700000000000273, -0.20799999999997, -0.20799999999997, -0.20799999999997, -0.20799999999997, -0.20799999999997, -0.20799999999997, -0.19800000000003593, -0.19800000000003593, -0.19800000000003593, -0.19800000000003593, -0.19400000000001683, -0.19400000000001683, -0.19400000000001683, -0.19400000000001683, -0.19400000000001683, -0.18799999999998818, -0.18799999999998818, -0.18799999999998818, -0.18799999999998818, -0.18799999999998818, -0.20099999999996498, -0.20099999999996498, -0.20099999999996498, -0.20099999999996498, -0.20099999999996498, -0.19800000000003593, -0.19800000000003593, -0.19800000000003593, -0.19800000000003593, 0.0, 0.0, 0.0, 0.0, 0.0, 0.0, 0.0, 0.0, 0.0, 0.0, 0.0, 0.0, 0.0, -0.21399999999999864, -0.21399999999999864, -0.21399999999999864, -0.19299999999998363, -0.19299999999998363, -0.19299999999998363], [2.799400340070858e-07, 2.799400340070858e-07, 2.799400340070858e-07, 2.799400340070858e-07, 4.8064628273461175e-09, 4.8064628273461175e-09, 4.8064628273461175e-09, 4.8064628273461175e-09, 4.8064628273461175e-09, 1.9272686950250605e-09, 1.9272686950250605e-09, 1.9272686950250605e-09, 1.9272686950250605e-09, 1.9272686950250605e-09, 7.744601902803624e-08, 7.744601902803624e-08, 7.744601902803624e-08, 7.744601902803624e-08, 7.744601902803624e-08, 4.962359157919599e-08, 4.962359157919599e-08, 4.962359157919599e-08, 4.962359157919599e-08, 4.962359157919599e-08, 3.267553601430304e-07, 3.267553601430304e-07, 3.267553601430304e-07, 3.267553601430304e-07, 3.267553601430304e-07, 4.998409103585882e-09, 4.998409103585882e-09, 4.998409103585882e-09, 4.998409103585882e-09, 4.998409103585882e-09, 4.4406565700798194e-08, 4.4406565700798194e-08, 4.4406565700798194e-08, 4.4406565700798194e-08, 4.4406565700798194e-08, 4.5095616003221444e-08, 4.5095616003221444e-08, 4.5095616003221444e-08, 4.5095616003221444e-08, 4.5095616003221444e-08, -2.500693197069776e-07, -2.500693197069776e-07, -2.500693197069776e-07, -2.500693197069776e-07, -2.500693197069776e-07, 6.405403841501323e-08, 6.405403841501323e-08, 6.405403841501323e-08, 6.405403841501323e-08]} caption="XY Graph"
  out "T_Cu (K)":dbl=286.483
  out "T_He (K)":dbl=286.676
  out "V (V)":dbl=0.00945189105599304 format="%_6g"
  out "I (A)":dbl=6.776848996201591e-06
  in  "Refresh boiling curve":bool
  out "Array dT":dbl[](array[numeric])=[-0.19700000000000273, -0.19700000000000273, -0.19700000000000273, -0.19700000000000273, -0.19700000000000273, -0.20799999999997, -0.20799999999997, -0.20799999999997, -0.20799999999997, -0.20799999999997, -0.20799999999997, -0.19800000000003593, -0.19800000000003593, -0.19800000000003593, -0.19800000000003593, -0.19400000000001683, -0.19400000000001683, -0.19400000000001683, -0.19400000000001683, -0.19400000000001683, -0.18799999999998818, -0.18799999999998818, -0.18799999999998818, -0.18799999999998818, -0.18799999999998818, -0.20099999999996498, -0.20099999999996498, -0.20099999999996498, -0.20099999999996498, -0.20099999999996498, -0.19800000000003593, -0.19800000000003593, -0.19800000000003593, -0.19800000000003593, 0.0, 0.0, 0.0, 0.0, 0.0, 0.0, 0.0, 0.0, 0.0, 0.0, 0.0, 0.0, 0.0, -0.21399999999999864, -0.21399999999999864, -0.21399999999999864, -0.19299999999998363, -0.19299999999998363]
  out "Array Q":dbl[](array[numeric])=[2.799400340070858e-07, 2.799400340070858e-07, 2.799400340070858e-07, 2.799400340070858e-07, 4.8064628273461175e-09, 4.8064628273461175e-09, 4.8064628273461175e-09, 4.8064628273461175e-09, 4.8064628273461175e-09, 1.9272686950250605e-09, 1.9272686950250605e-09, 1.9272686950250605e-09, 1.9272686950250605e-09, 1.9272686950250605e-09, 7.744601902803624e-08, 7.744601902803624e-08, 7.744601902803624e-08, 7.744601902803624e-08, 7.744601902803624e-08, 4.962359157919599e-08, 4.962359157919599e-08, 4.962359157919599e-08, 4.962359157919599e-08, 4.962359157919599e-08, 3.267553601430304e-07, 3.267553601430304e-07, 3.267553601430304e-07, 3.267553601430304e-07, 3.267553601430304e-07, 4.998409103585882e-09, 4.998409103585882e-09, 4.998409103585882e-09, 4.998409103585882e-09, 4.998409103585882e-09, 4.4406565700798194e-08, 4.4406565700798194e-08, 4.4406565700798194e-08, 4.4406565700798194e-08, 4.4406565700798194e-08, 4.5095616003221444e-08, 4.5095616003221444e-08, 4.5095616003221444e-08, 4.5095616003221444e-08, 4.5095616003221444e-08, -2.500693197069776e-07, -2.500693197069776e-07, -2.500693197069776e-07, -2.500693197069776e-07, -2.500693197069776e-07, 6.405403841501323e-08, 6.405403841501323e-08, 6.405403841501323e-08]
  out "Array time":dbl[](array[numeric])=[3667349477.3218102, 3667349477.5215826, 3667349477.721548, 3667349477.923008, 3667349478.1234393, 3667349478.3249006, 3667349478.524117, 3667349478.7243686, 3667349478.9248514, 3667349479.125014, 3667349479.3248487, 3667349479.5244465, 3667349479.7241926, 3667349479.9241066, 3667349480.124344, 3667349480.324479, 3667349480.524879, 3667349480.7243466, 3667349480.9258065, 3667349481.1252728, 3667349481.325767, 3667349481.525233, 3667349481.725702, 3667349481.925167, 3667349482.125595, 3667349482.3270874, 3667349482.5265527, 3667349482.7279825, 3667349482.9274473, 3667349483.127913, 3667349483.327517, 3667349483.5280623, 3667349483.727945, 3667349483.927341, 3667349484.1272106, 3667349484.3290305, 3667349484.528604, 3667349484.730065, 3667349484.9293137, 3667349485.130432, 3667349485.330589, 3667349485.5308065, 3667349485.7314234, 3667349485.9321766, 3667349486.1324425, 3667349486.3340607, 3667349486.5335255, 3667349486.734953, 3667349486.9344215, 3667349487.1351047, 3667349487.3345785, 3667349487.5342546]
  in  "BC file comment":string="Cu_flat_RUN4"
  out "Graph V SET":cluster{dbl[], dbl[]}(graph) caption="XY Graph"
  out "P (W)":dbl=6.405403841501323e-08 format="%_3f"
  in  "Select LSI 218/336":bool caption="OK Button"
  out "LSI-U out 1":dbl[](array[numeric])=[286.694, 286.481, 0.0, 0.0, 0.0, 0.0, 0.0, 0.0] format="%_3f"
  out "Graph LSI-U 1":cluster{dbl[], dbl[]}[](graph)=[{[3667349478.0127354, 3667349479.0140834, 3667349480.0134497, 3667349481.013572, 3667349482.014925, 3667349483.014216, 3667349484.015578, 3667349485.016135, 3667349486.016583, 3667349487.0163903, 3667349488.0179815, 3667349489.018835, 3667349490.018664, 3667349491.0187654, 3667349492.0187993, 3667349493.019667, 3667349494.019672, 3667349495.0196695, 3667349496.019436, 3667349497.021096, 3667349498.0206184], [286.686, 286.687, 286.675, 286.658, 286.691, 286.677, 286.684, 286.675, 286.697, 286.676, 286.678, 286.689, 286.65, 286.678, 286.665, 286.672, 286.658, 286.692, 286.701, 286.671, 286.694]}, {[3667349478.0127354, 3667349479.0140834, 3667349480.0134497, 3667349481.013572, 3667349482.014925, 3667349483.014216, 3667349484.015578, 3667349485.016135, 3667349486.016583, 3667349487.0163903, 3667349488.0179815, 3667349489.018835, 3667349490.018664, 3667349491.0187654, 3667349492.0187993, 3667349493.019667, 3667349494.019672, 3667349495.0196695, 3667349496.019436, 3667349497.021096, 3667349498.0206184], [286.478, 286.489, 286.481, 286.47, 286.49, 286.479, 286.483, 286.486, 286.483, 286.483, 286.488, 286.481, 286.476, 286.483, 286.477, 286.484, 286.48, 286.487, 286.476, 286.48, 286.481]}, {[3667349478.0127354, 3667349479.0140834, 3667349480.0134497, 3667349481.013572, 3667349482.014925, 3667349483.014216, 3667349484.015578, 3667349485.016135, 3667349486.016583, 3667349487.0163903, 3667349488.0179815, 3667349489.018835, 3667349490.018664, 3667349491.0187654, 3667349492.0187993, 3667349493.019667, 3667349494.019672, 3667349495.0196695, 3667349496.019436, 3667349497.021096, 3667349498.0206184], [0.0, 0.0, 0.0, 0.0, 0.0, 0.0, 0.0, 0.0, 0.0, 0.0, 0.0, 0.0, 0.0, 0.0, 0.0, 0.0, 0.0, 0.0, 0.0, 0.0, 0.0]}, {[3667349478.0127354, 3667349479.0140834, 3667349480.0134497, 3667349481.013572, 3667349482.014925, 3667349483.014216, 3667349484.015578, 3667349485.016135, 3667349486.016583, 3667349487.0163903, 3667349488.0179815, 3667349489.018835, 3667349490.018664, 3667349491.0187654, 3667349492.0187993, 3667349493.019667, 3667349494.019672, 3667349495.0196695, 3667349496.019436, 3667349497.021096, 3667349498.0206184], [0.0, 0.0, 0.0, 0.0, 0.0, 0.0, 0.0, 0.0, 0.0, 0.0, 0.0, 0.0, 0.0, 0.0, 0.0, 0.0, 0.0, 0.0, 0.0, 0.0, 0.0]}, {[3667349478.0127354, 3667349479.0140834, 3667349480.0134497, 3667349481.013572, 3667349482.014925, 3667349483.014216, 3667349484.015578, 3667349485.016135, 3667349486.016583, 3667349487.0163903, 3667349488.0179815, 3667349489.018835, 3667349490.018664, 3667349491.0187654, 3667349492.0187993, 3667349493.019667, 3667349494.019672, 3667349495.0196695, 3667349496.019436, 3667349497.021096, 3667349498.0206184], [0.0, 0.0, 0.0, 0.0, 0.0, 0.0, 0.0, 0.0, 0.0, 0.0, 0.0, 0.0, 0.0, 0.0, 0.0, 0.0, 0.0, 0.0, 0.0, 0.0, 0.0]}, {[3667349478.0127354, 3667349479.0140834, 3667349480.0134497, 3667349481.013572, 3667349482.014925, 3667349483.014216, 3667349484.015578, 3667349485.016135, 3667349486.016583, 3667349487.0163903, 3667349488.0179815, 3667349489.018835, 3667349490.018664, 3667349491.0187654, 3667349492.0187993, 3667349493.019667, 3667349494.019672, 3667349495.0196695, 3667349496.019436, 3667349497.021096, 3667349498.0206184], [0.0, 0.0, 0.0, 0.0, 0.0, 0.0, 0.0, 0.0, 0.0, 0.0, 0.0, 0.0, 0.0, 0.0, 0.0, 0.0, 0.0, 0.0, 0.0, 0.0, 0.0]}, {[3667349478.0127354, 3667349479.0140834, 3667349480.0134497, 3667349481.013572, 3667349482.014925, 3667349483.014216, 3667349484.015578, 3667349485.016135, 3667349486.016583, 3667349487.0163903, 3667349488.0179815, 3667349489.018835, 3667349490.018664, 3667349491.0187654, 3667349492.0187993, 3667349493.019667, 3667349494.019672, 3667349495.0196695, 3667349496.019436, 3667349497.021096, 3667349498.0206184], [0.0, 0.0, 0.0, 0.0, 0.0, 0.0, 0.0, 0.0, 0.0, 0.0, 0.0, 0.0, 0.0, 0.0, 0.0, 0.0, 0.0, 0.0, 0.0, 0.0, 0.0]}, {[3667349478.0127354, 3667349479.0140834, 3667349480.0134497, 3667349481.013572, 3667349482.014925, 3667349483.014216, 3667349484.015578, 3667349485.016135, 3667349486.016583, 3667349487.0163903, 3667349488.0179815, 3667349489.018835, 3667349490.018664, 3667349491.0187654, 3667349492.0187993, 3667349493.019667, 3667349494.019672, 3667349495.0196695, 3667349496.019436, 3667349497.021096, 3667349498.0206184], [0.0, 0.0, 0.0, 0.0, 0.0, 0.0, 0.0, 0.0, 0.0, 0.0, 0.0, 0.0, 0.0, 0.0, 0.0, 0.0, 0.0, 0.0, 0.0, 0.0, 0.0]}, {[3667349478.0127354, 3667349479.0140834, 3667349480.0134497, 3667349481.013572, 3667349482.014925, 3667349483.014216, 3667349484.015578, 3667349485.016135, 3667349486.016583, 3667349487.0163903, 3667349488.0179815, 3667349489.018835, 3667349490.018664, 3667349491.0187654, 3667349492.0187993, 3667349493.019667, 3667349494.019672, 3667349495.0196695, 3667349496.019436, 3667349497.021096, 3667349498.0206184], []}] caption="XY Graph"
  in  "log/linear 5":bool
  in  "Main loop\nWait (ms)":i32=1000
  in  "stop":bool
  out "current time":timestamp=timestamp(3667349498.0206184 s since 1904-01-01)
  out "Cycle #":i32=20
  in  "CSV filename suffix":string="test"
  in  "base path":path=path "C:/Users/TUCAN_rcnp/Desktop/Labview/TEST"
  out "ref LSI-U":refnum<file>
  out "ref DAQ":refnum<file>
  out "date/time string":string="20200318_131117_"
  out "ref LSI-D":refnum<file>
  out "ref RAW":refnum<file>
  # "LSI VISA addresses"
  # "Defines # of measurements \n taken for averaging\n (only tested with 5!)"
  # "NI DAQ OUT"
  # "LSI-336"
  # "LSI-218"
  # "DAQ OUT"
  # "DAQ OUT"
  # "MANUAL CTL"
  # "AUTO CTL"
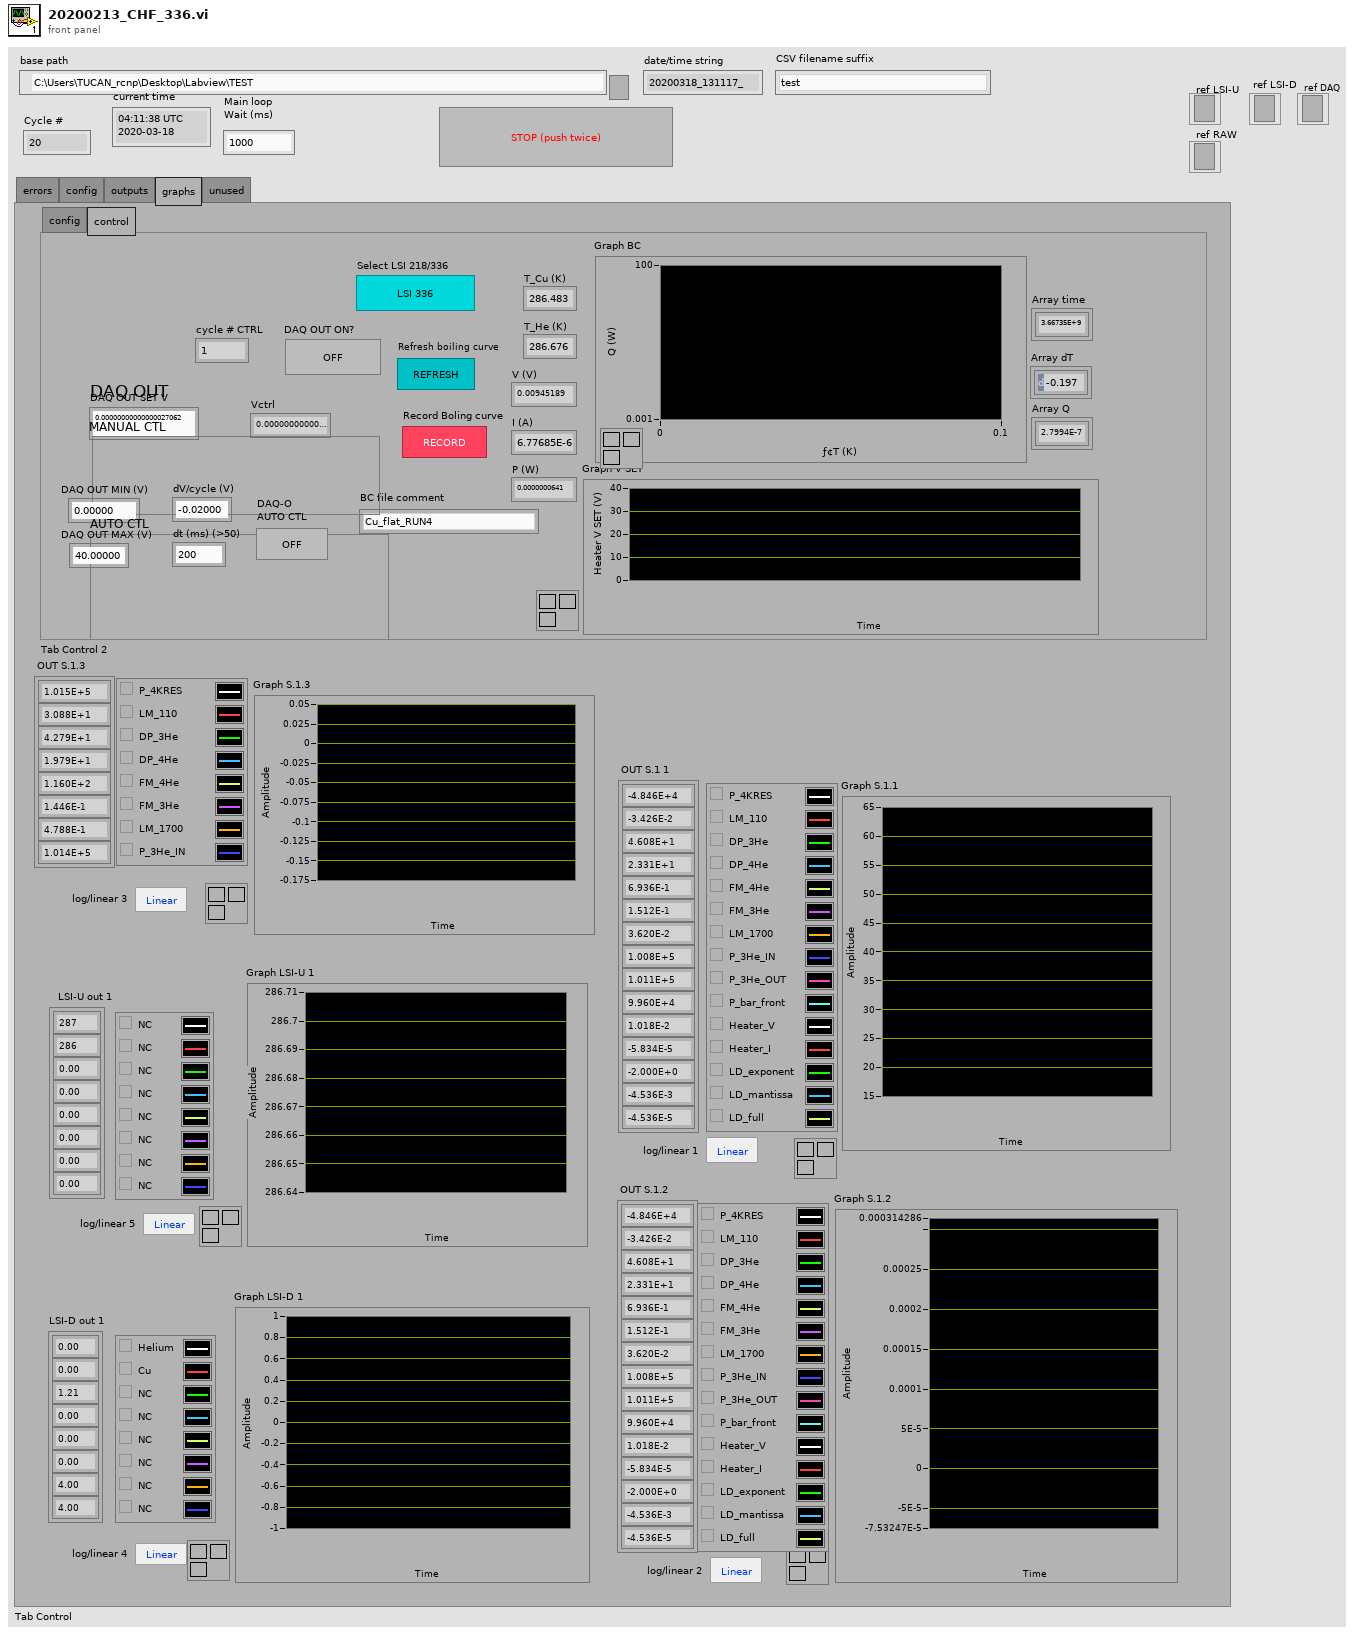
[diagram p1: front panel]
types:
  T1 = enum32{"errors", "config", "outputs", "graphs", "unused"}
  T2 = enum16{"open", "replace", "create", "open or create", "replace or create", "replace or create with confirmation"}
  T3 = cluster{"LSI-U CH labels[0]":string, "LSI-U CH labels[1]":string, "LSI-U CH labels[2]":string, "LSI-U CH labels[3]":string, "LSI-U CH labels[4]":string, "LSI-U CH labels[5]":string, "LSI-U CH labels[6]":string, "LSI-U CH labels[7]":string, "LSI-U CH labels[8]":string}
  T4 = cluster{"LSI-D CH labels[0]":string, "LSI-D CH labels[1]":string, "LSI-D CH labels[2]":string, "LSI-D CH labels[3]":string, "LSI-D CH labels[4]":string, "LSI-D CH labels[5]":string, "LSI-D CH labels[6]":string, "LSI-D CH labels[7]":string, "LSI-D CH labels[8]":string}
  T5 = cluster{"LSI-U out[0]":dbl, "LSI-U out[1]":dbl, "LSI-U out[2]":dbl, "LSI-U out[3]":dbl, "LSI-U out[4]":dbl, "LSI-U out[5]":dbl, "LSI-U out[6]":dbl, "LSI-U out[7]":dbl, "LSI-U out[8]":dbl}
  T6 = cluster{"LSI-D out[0]":dbl, "LSI-D out[1]":dbl, "LSI-D out[2]":dbl, "LSI-D out[3]":dbl, "LSI-D out[4]":dbl, "LSI-D out[5]":dbl, "LSI-D out[6]":dbl, "LSI-D out[7]":dbl, "LSI-D out[8]":dbl}
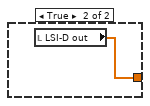
[diagram p2: hidden frame]
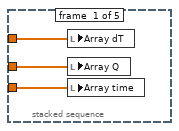
[diagram p3: hidden frame]
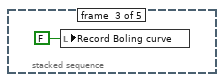
[diagram p5: hidden frame]
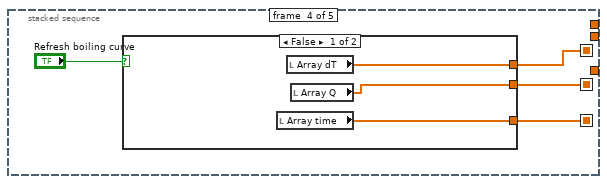
[diagram p6: hidden frame]
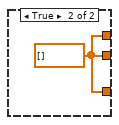
[diagram p7: hidden frame]
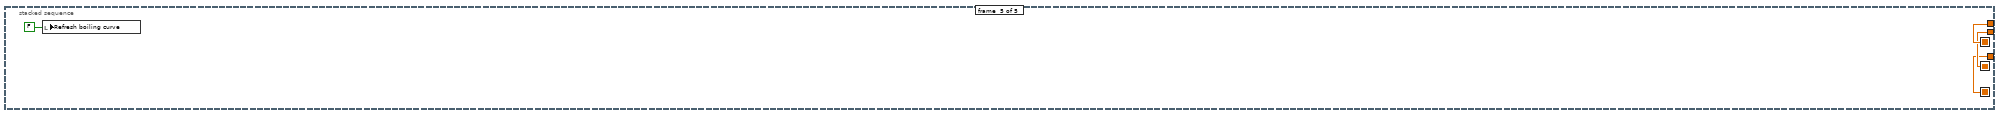
[diagram p8: hidden frame]
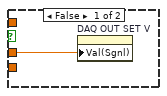
[diagram p10: hidden frame]
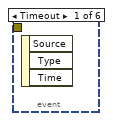
[diagram p11: hidden frame]
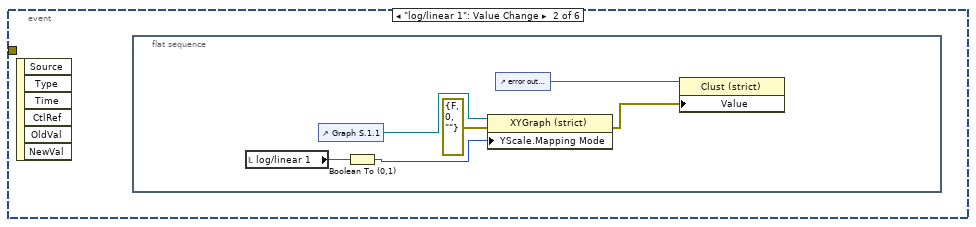
[diagram p12: hidden frame]
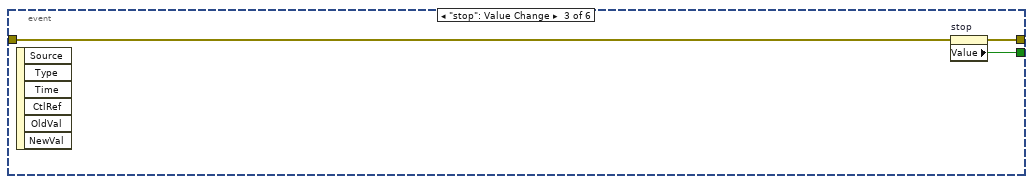
[diagram p13: hidden frame]
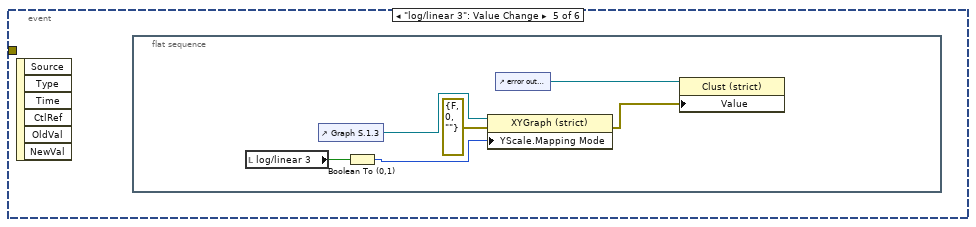
[diagram p14: hidden frame]
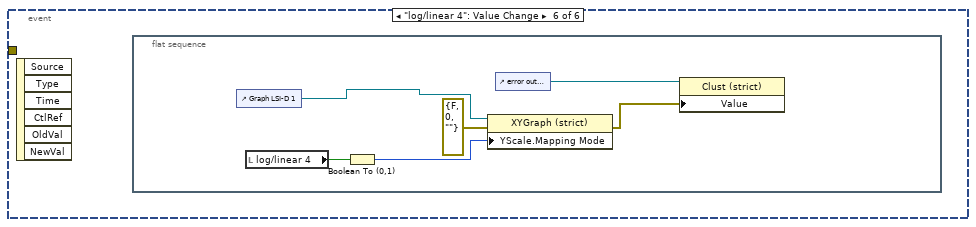
[diagram p15: hidden frame]
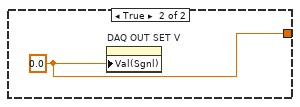
[diagram p16: hidden frame]
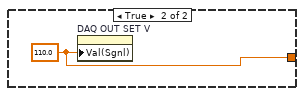
[diagram p17: hidden frame]
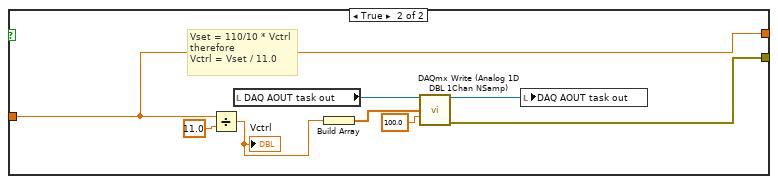
[diagram p18: hidden frame]
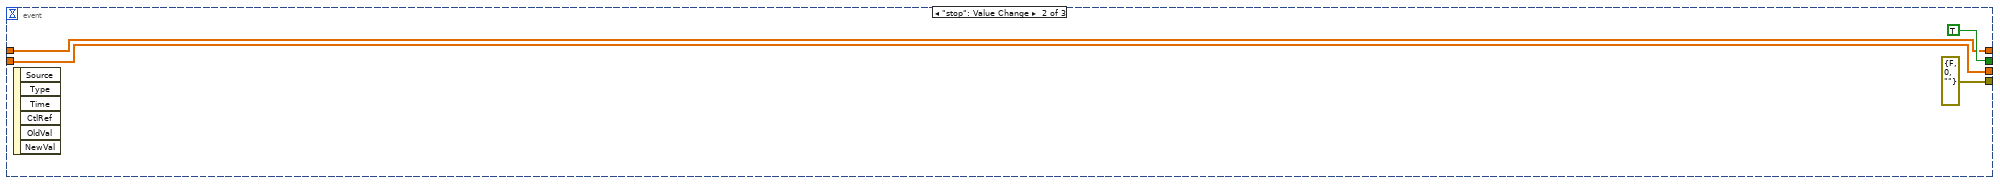
[diagram p19: hidden frame]
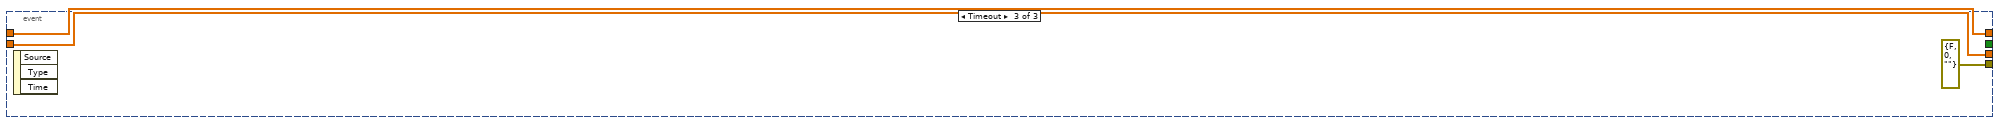
[diagram p20: hidden frame]
diagram:
  w5 = dbl[] []
  w9 = dbl[] []
  n1 = stacked-sequence {
    tunnel: [_ w151] -> w18
    tunnel: [_ w150] -> w34
    frame #0 {
      w57 = errorcluster {"status"=FALSE, "code"=0, "source"=""} ("error in")
      w52 = ".csv" ("string")
      w39 = T2."create" ("operation (0:open)")
      n2 = flat-sequence {
        frame #0 {
          (unwired) string[] ["Q1", "Q2", "Q3", "Q4", "Q5", "Q6", "Q7", "Q8", "Q9", "Q10", "Q11", "Q12"] ("DAQ CH")
          (unwired) string[] ["D1", "D2", "D3", "D4", "D5", "D6", "D7", "D8"] ("LSI-D CH")
          (unwired) string[] ["U1", "U2", "U3", "U4", "U5", "U6", "U7", "U8"] ("LSI-U CH 3")
          (unwired) i32[] [0, 1, 2, 3, 4, 5, 6, 7] ("idx in")
          (unwired) i32[] [0, 1, 2, 3, 4, 5, 6, 7, 8, 9, 10, 11] ("Q idx 2")
          # "CONSTANTS"
        }
      }
      n3 = Get Date/Time In Seconds() -> (seconds since 1Jan1904=w65:timestamp)
      n4 = Format Date/Time String(time format string (%c)="%Y%m%d_%H%M%S_", seconds (now)=w65) -> (date/time string=w43:string)  [unwired: 1 in]
      "date/time string" <- w43
      n5 = Concatenate Strings(w43, "CSV filename suffix", "_DAQ_RAW" ("string"), ".csv" ("string")) -> (w40:string)
      n6 = Concatenate Strings(w43, "CSV filename suffix", "_LSI336" ("string"), w52) -> (w62:string)
      n7 = Concatenate Strings(w43, "CSV filename suffix", "_LSI218" ("string"), w52) -> (w51:string)
      n8 = Concatenate Strings(w43, "CSV filename suffix", "_DAQ" ("string"), w52) -> (w60:string)
      n9 = Build Path(base path="base path", name or relative path=w40) -> (appended path=w38:path)
      n10 = Build Path(base path="base path", name or relative path=w62) -> (appended path=w63:path)
      n11 = Build Path(base path="base path", name or relative path=w51) -> (appended path=w50:path)
      n12 = Build Path(base path="base path", name or relative path=w60) -> (appended path=w58:path)
      n13 = Open/Create/Replace File(file path (use dialog)=w63, error in=w57, operation (0:open)=w39) -> (refnum out=w56:refnum<file>)  [unwired: 3 in, 2 out]
      "ref LSI-U" <- w56
      n14 = Open/Create/Replace File(file path (use dialog)=w58, error in=w57, operation (0:open)=w39) -> (refnum out=w55:refnum<file>, error out=w49:errorcluster)  [unwired: 3 in, 1 out]
      "ref DAQ" <- w55
      n15 = Open/Create/Replace File(file path (use dialog)=w50, error in=w49, operation (0:open)=w39) -> (refnum out=w46:refnum<file>, error out=w37:errorcluster)  [unwired: 3 in, 1 out]
      "ref LSI-D" <- w46
      n16 = Open/Create/Replace File(file path (use dialog)=w38, error in=w37, operation (0:open)=w39) -> (refnum out=w35:refnum<file>, error out=w36:errorcluster)  [unwired: 3 in, 1 out]
      "ref RAW" <- w35
      n17 = flat-sequence {
        tunnel: w56 -> [w82]
        tunnel: w36 -> [w81]
        tunnel: [w77] -> w48
        tunnel: w48 -> [w87]
        tunnel: [w86] -> w47
        tunnel: w46 -> [w85]
        tunnel: w47 -> [w105]
        tunnel: w55 -> [w104]
        tunnel: [w103] -> w54
        tunnel: w35 -> [w102]
        frame #0 {
          # "Write the column names"
          n18 = local read "LSI-U CH labels"() -> (w75:string[])
          n19 = Array To Cluster(array=w75) -> (cluster=w74:T3)
          n20 = Unbundle(w74) -> ("LSI-U CH labels[0]"=w73:string, "LSI-U CH labels[1]"=w72:string, "LSI-U CH labels[2]"=w71:string, "LSI-U CH labels[3]"=w70:string, "LSI-U CH labels[4]"=w69:string, "LSI-U CH labels[5]"=w68:string, "LSI-U CH labels[6]"=w67:string, "LSI-U CH labels[7]"=w66:string)  [unwired: 1 out]
          n21 = Format Into String(format string="%s,%s,%s,%s,%s,%s,%s,%s,%s,%s,%s,%s\\n" ("time format string (%c)"), initial string=w82, error in=w81, "INDEX" ("input 1"), "Datetime" ("input 1"), "UNIX_time" ("input 1"), "LV_time" ("input 1"), w73, w72, w71, w70, w69, w68, w67, w66) -> (error out=w77:errorcluster)  [unwired: 1 out]
        }
        frame #1 {
          # "Write the column names"
          n22 = local read "LSI-D CH labels"() -> (w92:string[])
          n23 = Array To Cluster(array=w92) -> (cluster=w93:T4)
          n24 = Unbundle(w93) -> ("LSI-D CH labels[0]"=w94:string, "LSI-D CH labels[1]"=w95:string, "LSI-D CH labels[2]"=w96:string, "LSI-D CH labels[3]"=w97:string, "LSI-D CH labels[4]"=w98:string, "LSI-D CH labels[5]"=w99:string, "LSI-D CH labels[6]"=w100:string, "LSI-D CH labels[7]"=w101:string)  [unwired: 1 out]
          n25 = Format Into String(format string="%s,%s,%s,%s,%s,%s,%s,%s,%s,%s,%s,%s\\n" ("time format string (%c)"), initial string=w85, error in=w87, "INDEX" ("input 1"), "Datetime" ("input 1"), "UNIX_time" ("input 1"), "LV_time" ("input 1"), w94, w95, w96, w97, w98, w99, w100, w101) -> (error out=w86:errorcluster)  [unwired: 1 out]
        }
        frame #2 {
          n26 = stacked-sequence {
            tunnel: w105 -> [w122 w142]
            tunnel: w104 -> [w121 _]
            tunnel: [w120 _] -> w103
            tunnel: w102 -> [_ w128]
            frame #0 {
              # "Write the column names"
              n27 = local read "DAQ-AIN labels"() -> (w118:string[])
              n28 = Index Array(array=w118) -> (element #1=w117:string, element #2=w116:string, element #3=w115:string, element #4=w114:string, element #5=w112:string, element #6=w113:string, element #7=w111:string, element #8=w110:string, element #9=w109:string, element #10=w108:string, element #11=w107:string, element #12=w106:string)  [unwired: 13 in, 1 out]
              n29 = Format Into String(format string="%s,%s,%s,%s,%s,%s,%s,%s,%s,%s,%s,%s,%s,%s,%s,%s\\n" ("time format string (%c)"), initial string=w121, error in=w122, "INDEX" ("input 1"), "Datetime" ("input 1"), "UNIX_time" ("input 1"), "LV_time" ("input 1"), w117, w116, w115, w114, w112, w113, w111, w110, w109, w108, w107, w106) -> (error out=w120:errorcluster)  [unwired: 1 out]
            }
            frame #1 {
              # "Write the column names"
              n30 = local read "DAQ-AIN labels"() -> (w140:string[])
              n31 = Index Array(array=w140) -> (element #1=w139:string, element #2=w138:string, element #3=w137:string, element #4=w136:string, element #5=w134:string, element #6=w135:string, element #7=w133:string, element #8=w132:string, element #9=w131:string, element #10=w130:string, element #11=w129:string, element #12=w127:string)  [unwired: 12 in]
              n32 = Format Into String(format string="%s,%s,%s,%s,%s,%s,%s,%s,%s,%s,%s,%s,%s,%s,%s,%s\\n" ("time format string (%c)"), initial string=w128, error in=w142, "INDEX" ("input 1"), "Datetime" ("input 1"), "UNIX_time" ("input 1"), "LV_time" ("input 1"), w139, w138, w137, w136, w134, w135, w133, w132, w131, w130, w129, w127) -> ()  [unwired: 2 out]
            }
          }
        }
      }
      "error out\n(file creation)" <- w54
    }
    frame #1 {
      # "DAQ config"
      n33 = feedback #1() -> (w147:errorcluster)  [unwired: 1 in]
      n34 = stacked-sequence {
        tunnel: [w152 _] -> w148
        tunnel: [w153 _] -> w151
        tunnel: [_ w187] -> w150
        tunnel: [_ w186] -> w149
        tunnel: w147 -> [_ w180]
        frame #0 {
          # "read task"
          n35 = local read "date/time string"() -> (w163:string)
          n36 = Concatenate Strings(w163, "AI" ("new task name")) -> (w161:string)
          n37 = call <vilib>:"DAQmx Create Task.vi"("new task name"=w161, "error in"=errorcluster {"status"=FALSE, "code"=0, "source"=""}) -> ("task out"=w159:refnum<k21>, "error out"=w160:errorcluster)  [unwired: 12 in]
          n38 = for {
            shift-right: [w172] -> w154
            shift-left: w160 -> [w171]
            shift-right: [w170] -> w155
            shift-left: w159 -> [w169]
            tunnel: "DAQ AIN channels" -> [w168] mode=indexing
            tunnel: "V_min(in)" -> [w167] mode=indexing
            tunnel: "V_max(in)" -> [w166] mode=indexing
            w165 = 10106 items=["Default"=-1, "RSE"=10083, "NRSE"=10078, "Differential"=10106, "Pseudodifferential"=12529] ("input terminal configuration")
            n39 = call-poly <vilib>:"DAQmx Create Virtual Channel.vi"("task in"=w169, "maximum value"=w166, "minimum value"=w167, "input terminal configuration"=w165, "physical channels"=w168, "error in"=w171) -> ("task out"=w170:refnum<k21>, "error out"=w172:errorcluster)  [unwired: 8 in]
          }
          n40 = call <vilib>:"DAQmx Start Task.vi"("task/channels in"=w155, "error in"=w154) -> ("task out"=w153:refnum<k21>, "error out"=w152:errorcluster)  [unwired: 12 in]
        }
        frame #1 {
          w177 = -1 items=["Default"=-1, "RSE"=10083, "Differential"=10106, "Pseudodifferential"=12529] ("output terminal configuration")
          w176 = 10348 items=["Volts"=10348, "From Custom Scale"=10065] ("units")
          # "write task"
          n41 = local read "date/time string"() -> (w183:string)
          n42 = Concatenate Strings(w183, "AO" ("new task name")) -> (w181:string)
          n43 = call <vilib>:"DAQmx Create Task.vi"("new task name"=w181, "error in"=w180) -> ("task out"=w185:refnum<k21>, "error out"=w184:errorcluster)  [unwired: 12 in]
          n44 = call-poly <vilib>:"DAQmx Create Virtual Channel.vi"("task in"=w185, "maximum value"="V_lim_max", "minimum value"="V_lim_min", "output terminal configuration"=w177, "physical channels"="DAQ AOUT ch", "units"=w176, "error in"=w184) -> ("task out"=w179:refnum<k21>, "error out"=w178:errorcluster)  [unwired: 7 in]
          n45 = call <vilib>:"DAQmx Start Task.vi"("task/channels in"=w179, "error in"=w178) -> ("task out"=w187:refnum<k21>, "error out"=w186:errorcluster)  [unwired: 12 in]
        }
      }
      "error out\n(DAQ config)" <- w149
      n46 = feedback-in #1(w148) -> ()
    }
  }
  "DAQ AOUT task out" <- w34
  "DAQ AIN task out" <- w18
  n47 = invoke on="DAQ OUT ON?" class="Bool (strict)" method="Reinit To Default"(error in=errorcluster {"status"=FALSE, "code"=0, "source"=""} ("error in (no error)")) -> (error out=w13:errorcluster)  [unwired: 2 in, 2 out]
  n48 = invoke on="DAQ-O \nAUTO CTL" class="Bool (strict)" method="Reinit To Default"(error in=w13) -> (error out=w12:errorcluster)  [unwired: 2 in, 2 out]
  n49 = invoke on="stop" class="Bool (strict)" method="Reinit To Default"(error in=w12) -> (error out=w6:errorcluster)  [unwired: 2 in, 2 out]
  n50 = call "Initialize.vi"("error in (no error)"=errorcluster {"status"=FALSE, "code"=0, "source"=""}, "VISA resource name"="VISA LSI336") -> ("error out"=w2:errorcluster, "VISA resource name out"=w3:refnum<visa-resource-name>)  [unwired: 8 in]
  n51 = call "Initialize.vi"("VISA resource name"="VISA LSI218 UP", "error in (no error)"=errorcluster {"status"=FALSE, "code"=0, "source"=""}) -> ("VISA resource name out"=w33:refnum<visa-resource-name>, "error out"=w32:errorcluster)  [unwired: 12 in]
  n52 = while {
    tunnel: w6 -> [w190]
    tunnel: [w189] -> w14
    stop <- w188 stop-if-true
    n53 = event shown="[3] \"log/linear 2\": Value Change" {
      selector: _ -> [_ _ _ _ _ _]
      dyn-events: _ -> [_ _ _ _ _ _]
      timeout: _ -> [_ _ _ _ _ _]
      tunnel: w190 -> [_ _ w200 _ _ _]
      tunnel: [_ _ w199 _ _ _] -> w189
      tunnel: [_ _ w198 _ _ _] -> w188
      event Timeout {
        n54 = event-data() -> ()  [unwired: 1 in, 3 out]
      }
      event "log/linear 1": Value Change {
        n55 = event-data() -> ()  [unwired: 1 in, 6 out]
        n56 = flat-sequence {
          frame #0 {
            n57 = local read "log/linear 1"() -> (w196:bool)
            n58 = control-ref of="Graph S.1.1"() -> (w193:refnum<vi>)
            n59 = Boolean To (0,1)(Boolean=w196) -> (0, 1=w195:i16)
            n60 = property class="XYGraph (strict)"(reference=w193, error in=errorcluster {"status"=FALSE, "code"=0, "source"=""} ("error in (no error)"), "YScale.Mapping Mode"=w195) -> (error out=w194:errorcluster)  [unwired: 1 out]
            n61 = control-ref of="error out (decoration)"() -> (w192:refnum<vi>)
            n62 = property class="Clust (strict)"(reference=w192, "Value"=w194) -> ()  [unwired: 1 in, 2 out]
          }
        }
      }
      event "stop": Value Change {
        n63 = event-data() -> ()  [unwired: 1 in, 6 out]
        n64 = property on="stop" class="Bool (strict)"(error in=w200) -> (error out=w199:errorcluster, "Value"=w198:bool)  [unwired: 1 in, 1 out]
      }
      event "log/linear 2": Value Change {
        n65 = event-data() -> ()  [unwired: 1 in, 6 out]
        n66 = flat-sequence {
          frame #0 {
            n67 = local read "log/linear 2"() -> (w203:bool)
            n68 = control-ref of="Graph S.1.2"() -> (w202:refnum<vi>)
            n69 = Boolean To (0,1)(Boolean=w203) -> (0, 1=w205:i16)
            n70 = property class="XYGraph (strict)"(reference=w202, error in=errorcluster {"status"=FALSE, "code"=0, "source"=""} ("error in (no error)"), "YScale.Mapping Mode"=w205) -> (error out=w204:errorcluster)  [unwired: 1 out]
            n71 = control-ref of="error out (decoration)"() -> (w201:refnum<vi>)
            n72 = property class="Clust (strict)"(reference=w201, "Value"=w204) -> ()  [unwired: 1 in, 2 out]
          }
        }
      }
      event "log/linear 3": Value Change {
        n73 = event-data() -> ()  [unwired: 1 in, 6 out]
        n74 = flat-sequence {
          frame #0 {
            n75 = local read "log/linear 3"() -> (w209:bool)
            n76 = control-ref of="Graph S.1.3"() -> (w207:refnum<vi>)
            n77 = Boolean To (0,1)(Boolean=w209) -> (0, 1=w211:i16)
            n78 = property class="XYGraph (strict)"(reference=w207, error in=errorcluster {"status"=FALSE, "code"=0, "source"=""} ("error in (no error)"), "YScale.Mapping Mode"=w211) -> (error out=w210:errorcluster)  [unwired: 1 out]
            n79 = control-ref of="error out (decoration)"() -> (w208:refnum<vi>)
            n80 = property class="Clust (strict)"(reference=w208, "Value"=w210) -> ()  [unwired: 1 in, 2 out]
          }
        }
      }
      event "log/linear 4": Value Change {
        n81 = event-data() -> ()  [unwired: 1 in, 6 out]
        n82 = flat-sequence {
          frame #0 {
            n83 = control-ref of="Graph LSI-D 1"() -> (w213:refnum<vi>)
            n84 = local read "log/linear 4"() -> (w215:bool)
            n85 = Boolean To (0,1)(Boolean=w215) -> (0, 1=w217:i16)
            n86 = property class="XYGraph (strict)"(reference=w213, error in=errorcluster {"status"=FALSE, "code"=0, "source"=""} ("error in (no error)"), "YScale.Mapping Mode"=w217) -> (error out=w216:errorcluster)  [unwired: 1 out]
            n87 = control-ref of="error out (decoration)"() -> (w214:refnum<vi>)
            n88 = property class="Clust (strict)"(reference=w214, "Value"=w216) -> ()  [unwired: 1 in, 2 out]
          }
        }
      }
    }
    n89 = Wait (ms)(milliseconds to wait=u32 300) -> ()  [unwired: 1 out]
  }
  n90 = while {
    shift-right: [w234] -> _
    shift-left: dbl[] [] -> [w243]
    shift-right: [w237] -> _
    shift-left: dbl[][] [] -> [w238]
    shift-right: [w233] -> _
    shift-left: dbl[][] [] -> [w239]
    tunnel: [w232] -> w24
    shift-right: [w219] -> _
    shift-left: dbl[][] [] -> [w229]
    tunnel: w33 -> [w228]
    tunnel: w32 -> [w227]
    tunnel: w2 -> [w226]
    tunnel: w3 -> [w225]
    tunnel: [w224] -> w23
    tunnel: w18 -> [w222]
    tunnel: [w221] -> w16
    tunnel: w6 -> [w221]
    i -> [w240]
    stop <- w220 stop-if-true
    n91 = flat-sequence {
      frame #0 {
        n92 = local read "DAQ-AIN labels"() -> (→"DAQ AIN CH indic.":string[])
        n93 = local read "LSI-U CH labels"() -> (→"LSI-U CH indic,":string[])
        n94 = local read "LSI-D CH labels"() -> (→"LSI-D CH indic.":string[])
      }
    }
    n95 = property on="stop" class="Bool (strict)"(error in=w221) -> ("Value"=w220:bool)  [unwired: 1 in, 2 out]
    n96 = Get Date/Time In Seconds() -> (seconds since 1Jan1904=→"current time":timestamp)
    n97 = local read "current time"() -> (w241:timestamp)
    n98 = Wait (ms)(milliseconds to wait="Main loop\nWait (ms)") -> ()  [unwired: 1 out]
    n99 = To Double Precision Float(number=w241) -> (double precision float=w242:dbl)
    n100 = Build Array (concatenate)(w243, w242) -> (w234:dbl[])
    n101 = flat-sequence {
      tunnel: w234 -> [w565]
      tunnel: w238 -> [w597]
      tunnel: [w595] -> w235
      tunnel: [w566] -> w230
      tunnel: w229 -> [w567]
      tunnel: w228 -> [w561]
      tunnel: w227 -> [w560]
      tunnel: w226 -> [w557]
      tunnel: w225 -> [w556]
      tunnel: [w698] -> w236
      tunnel: w235 -> [w698]
      tunnel: [w697] -> w231
      tunnel: w230 -> [w697]
      tunnel: [w715] -> w237
      tunnel: w236 -> [w715]
      tunnel: [w710] -> w219
      tunnel: w231 -> [w710]
      frame #0 {
        n102 = call "Data Sensor.vi"("VISA resource name"=w561, "error in (no error)"=w560) -> ("Input 1"=w606:dbl, "Input 2"=w605:dbl, "Input 3"=w604:dbl, "VISA resource name out"=w598:refnum<visa-resource-name>, "Input 4"=w596:dbl, "Input 5"=w603:dbl, "Input 6"=w602:dbl, "Input 8"=w600:dbl, "Input 7"=w601:dbl, "error out"=w599:errorcluster)  [unwired: 4 in]
        n103 = case shown="True" TRUE {
          tunnel: w567 -> [w607 w630]
          tunnel: [w607 w629] -> w566
          tunnel: w565 -> [_ w628]
          tunnel: w557 -> [_ w625]
          tunnel: w556 -> [_ w626]
          frame False {
          }
          frame True {
            w608 = 0.0 ("element")
            n104 = flat-sequence {
              tunnel: w626 -> [w663]
              tunnel: w625 -> [w661]
              tunnel: [w663] -> w623
              tunnel: [w662] -> w622
              tunnel: [w659] -> w621
              tunnel: [w658] -> w614
              tunnel: w623 -> [w667]
              tunnel: w622 -> [_]
              tunnel: w621 -> [w665]
              tunnel: [w667] -> w620
              tunnel: [w665] -> w619
              tunnel: [w664] -> w613
              tunnel: w620 -> [w671]
              tunnel: [w671] -> w618
              tunnel: w619 -> [w670]
              tunnel: [w670] -> w617
              tunnel: [w668] -> w612
              tunnel: w618 -> [w677]
              tunnel: w617 -> [w676]
              tunnel: [w674] -> w616
              tunnel: [w673] -> w615
              tunnel: [w672] -> w611
              frame #0 {
                w660 = u16 0 items=["A", "B", "C", "D"] ("Input (0:A)")
                n105 = call-poly "Sensor Data.vi"("error in (no error)"=w661, "Input (0:A)"=w660, "VISA resource name"=w663) -> ("error out"=w659:errorcluster, "Sensor Data"=w658:dbl, "VISA resource name out"=w662:refnum<visa-resource-name>)  [unwired: 6 in]
              }
              frame #1 {
                w666 = u16 1 items=["A", "B", "C", "D"] ("Input (0:A)")
                n106 = call-poly "Sensor Data.vi"("error in (no error)"=w665, "Input (0:A)"=w666, "VISA resource name"=w667) -> ("Sensor Data"=w664:dbl)  [unwired: 6 in, 2 out]
              }
              frame #2 {
                w669 = u16 2 items=["A", "B", "C", "D"] ("Input (0:A)")
                n107 = call-poly "Sensor Data.vi"("error in (no error)"=w670, "Input (0:A)"=w669, "VISA resource name"=w671) -> ("Sensor Data"=w668:dbl)  [unwired: 6 in, 2 out]
              }
              frame #3 {
                w675 = u16 3 items=["A", "B", "C", "D"] ("Input (0:A)")
                n108 = call-poly "Sensor Data.vi"("error in (no error)"=w676, "Input (0:A)"=w675, "VISA resource name"=w677) -> ("error out"=w673:errorcluster, "Sensor Data"=w672:dbl, "VISA resource name out"=w674:refnum<visa-resource-name>)  [unwired: 6 in]
              }
            }
            n109 = control-ref of="error out (LSI)"() -> (w627:refnum<vi>)
            n110 = call "Close.vi"("error in (no error)"=w615, "VISA resource name"=w616) -> ("error out"=w624:errorcluster)  [unwired: 9 in]
            n111 = Build Array(w614, w613, w612, w611, w608, w608, w608, w608) -> (w610:dbl[])
            "LSI-U out" <- w610
            "LSI-U out 1" <- w610
            n112 = property class="Clust (strict)"(reference=w627, "Value"=w624) -> ()  [unwired: 1 in, 2 out]
            n113 = Build Array (concatenate)(w630, w610) -> (w629:dbl[][])
            n114 = Index Array(array=w629, index (col) #1=0 ("disabled index (col)"), index (col) #2=1 ("index (col)"), index (col) #3=2 ("index (col)"), index (col) #4=3 ("index (col)"), index (col) #5=4 ("index (col)"), index (col) #6=5 ("index (col)"), index (col) #7=6 ("index (col)"), index (col) #8=7 ("index (col)"), index (col) #9=8 ("index (col)")) -> (element #1=w632:dbl[], element #2=w641:dbl[], element #3=w642:dbl[], element #4=w643:dbl[], element #5=w644:dbl[], element #6=w645:dbl[], element #7=w646:dbl[], element #8=w647:dbl[], element #9=w648:dbl[])  [unwired: 9 in]
            n115 = Bundle(w628, w632) -> (w649:cluster{dbl[], dbl[]})  [unwired: 1 in]
            n116 = Bundle(w628, w641) -> (w650:cluster{dbl[], dbl[]})  [unwired: 1 in]
            n117 = Bundle(w628, w642) -> (w651:cluster{dbl[], dbl[]})  [unwired: 1 in]
            n118 = Bundle(w628, w643) -> (w652:cluster{dbl[], dbl[]})  [unwired: 1 in]
            n119 = Bundle(w628, w644) -> (w653:cluster{dbl[], dbl[]})  [unwired: 1 in]
            n120 = Bundle(w628, w645) -> (w654:cluster{dbl[], dbl[]})  [unwired: 1 in]
            n121 = Bundle(w628, w646) -> (w655:cluster{dbl[], dbl[]})  [unwired: 1 in]
            n122 = Bundle(w628, w647) -> (w656:cluster{dbl[], dbl[]})  [unwired: 1 in]
            n123 = Bundle(w628, w648) -> (w657:cluster{dbl[], dbl[]})  [unwired: 1 in]
            n124 = Build Array(w649, w650, w651, w652, w653, w654, w655, w656, w657) -> (w609:cluster{dbl[], dbl[]}[])
            n125 = local write "Graph LSI-U 1"(w609) -> ()
          }
        }
        n126 = call "Close.vi"("VISA resource name"=w598, "error in (no error)"=w599) -> ("error out"=w559:errorcluster)  [unwired: 13 in]
        n127 = Build Array(w606, w605, w604, w596, w603, w602, w601, w600) -> (w554:dbl[])
        "LSI-D out" <- w554
        "LSI-D out 1" <- w554
        n128 = control-ref of="error out (LSI)"() -> (w558:refnum<vi>)
        n129 = property class="Clust (strict)"(reference=w558, "Value"=w559) -> ()  [unwired: 1 in, 2 out]
        n130 = Build Array (concatenate)(w597, w554) -> (w595:dbl[][])
        n131 = Index Array(array=w595, index (col) #1=0 ("disabled index (col)"), index (col) #2=1 ("index (col)"), index (col) #3=2 ("index (col)"), index (col) #4=3 ("index (col)"), index (col) #5=4 ("index (col)"), index (col) #6=5 ("index (col)"), index (col) #7=6 ("index (col)"), index (col) #8=7 ("index (col)"), index (col) #9=8 ("index (col)")) -> (element #1=w593:dbl[], element #2=w584:dbl[], element #3=w583:dbl[], element #4=w582:dbl[], element #5=w581:dbl[], element #6=w580:dbl[], element #7=w579:dbl[], element #8=w578:dbl[], element #9=w577:dbl[])  [unwired: 9 in]
        n132 = Bundle(w565, w593) -> (w576:cluster{dbl[], dbl[]})  [unwired: 1 in]
        n133 = Bundle(w565, w584) -> (w575:cluster{dbl[], dbl[]})  [unwired: 1 in]
        n134 = Bundle(w565, w583) -> (w574:cluster{dbl[], dbl[]})  [unwired: 1 in]
        n135 = Bundle(w565, w582) -> (w573:cluster{dbl[], dbl[]})  [unwired: 1 in]
        n136 = Bundle(w565, w581) -> (w572:cluster{dbl[], dbl[]})  [unwired: 1 in]
        n137 = Bundle(w565, w580) -> (w571:cluster{dbl[], dbl[]})  [unwired: 1 in]
        n138 = Bundle(w565, w579) -> (w570:cluster{dbl[], dbl[]})  [unwired: 1 in]
        n139 = Bundle(w565, w578) -> (w569:cluster{dbl[], dbl[]})  [unwired: 1 in]
        n140 = Bundle(w565, w577) -> (w568:cluster{dbl[], dbl[]})  [unwired: 1 in]
        n141 = Build Array(w576, w575, w574, w573, w572, w571, w570, w569, w568) -> (w555:cluster{dbl[], dbl[]}[])
        n142 = local write "Graph LSI-D 1"(w555) -> ()
        n143 = feedback #2() -> (w563:errorcluster)  [unwired: 1 in]
        n144 = stacked-sequence {
          tunnel: [w680 _] -> w564
          tunnel: [_ w689] -> w562
          tunnel: w563 -> [_ w688]
          frame #0 {
            n145 = local read "LSI-D CH indic."() -> (w679:string[])
            n146 = control-ref of="Graph LSI-D 1"() -> (w678:refnum<vi>)
            n147 = Array Size(array=w679) -> (size(s)=w681:i32)
            n148 = for {
              N: w681 -> [_]
              tunnel: [w684] -> w680
              tunnel: w679 -> [w683] mode=indexing
              tunnel: w678 -> [w682]
              i -> [w685]
              n149 = property class="XYGraph (strict)"(reference=w682, error in=errorcluster {"status"=FALSE, "code"=0, "source"=""} ("error in (no error)"), "Active Plot"=w685, "Plot.Plot Name"=w683) -> (error out=w684:errorcluster)  [unwired: 1 out]
            }
          }
          frame #1 {
            n150 = local read "LSI-U CH indic,"() -> (w690:string[])
            n151 = control-ref of="Graph LSI-U 1"() -> (w687:refnum<vi>)
            n152 = Array Size(array=w690) -> (size(s)=w691:i32)
            n153 = for {
              N: w691 -> [_]
              tunnel: w690 -> [w695] mode=indexing
              tunnel: [w694] -> w689
              tunnel: w688 -> [w693]
              tunnel: w687 -> [w692]
              i -> [w696]
              n154 = property class="XYGraph (strict)"(reference=w692, error in=w693, "Active Plot"=w696, "Plot.Plot Name"=w695) -> (error out=w694:errorcluster)  [unwired: 1 out]
            }
          }
        }
        n155 = feedback-in #2(w564) -> ()
        n156 = control-ref of="error out (decoration)"() -> (w553:refnum<vi>)
        n157 = property class="Clust (strict)"(reference=w553, "Value"=w562) -> ()  [unwired: 1 in, 2 out]
      }
      frame #1 {
      }
      frame #2 {
        n158 = local read "LSI-D out"() -> (w709:dbl[])
        n159 = case shown="True" FALSE {
          frame False {
          }
          frame True {
            n160 = local read "LSI-U out"() -> (w728:dbl[])
            n161 = local read "current time"() -> (w732:timestamp)
            n162 = Array To Cluster(array=w728) -> (cluster=w731:T5)
            n163 = local read "ref LSI-U"() -> (w727:refnum<file>)
            n164 = local read "Cycle #"() -> (w735:i32)
            n165 = To Double Precision Float(number=w732) -> (double precision float=w729:dbl)
            n166 = call "LV_UNIX.vi"("current time"=w732) -> ("date/time string"=w734:string, "UNIX time (s)"=w733:dbl)  [unwired: 9 in]
            n167 = Unbundle(w731) -> ("LSI-U out[0]"=w724:dbl, "LSI-U out[1]"=w725:dbl, "LSI-U out[2]"=w726:dbl, "LSI-U out[3]"=w723:dbl, "LSI-U out[4]"=w722:dbl, "LSI-U out[5]"=w721:dbl, "LSI-U out[6]"=w720:dbl, "LSI-U out[7]"=w719:dbl)  [unwired: 1 out]
            n168 = Format Into String(format string="%d,%s,%10.4f,%10.4f,%5.6f,%5.6f,%5.6f,%5.6f,%5.6f,%5.6f,%5.6f,%5.6f\\n", initial string=w727, w735, w734, w733, w729, w724, w725, w726, w723, w722, w721, w720, w719) -> ()  [unwired: 1 in, 2 out]
          }
        }
        n169 = local read "current time"() -> (w714:timestamp)
        n170 = Array To Cluster(array=w709) -> (cluster=w716:T6)
        n171 = To Double Precision Float(number=w714) -> (double precision float=w718:dbl)
        n172 = call "LV_UNIX.vi"("current time"=w714) -> ("date/time string"=w712:string, "UNIX time (s)"=w713:dbl)  [unwired: 9 in]
        n173 = Unbundle(w716) -> ("LSI-D out[0]"=w707:dbl, "LSI-D out[1]"=w706:dbl, "LSI-D out[2]"=w705:dbl, "LSI-D out[3]"=w704:dbl, "LSI-D out[4]"=w703:dbl, "LSI-D out[5]"=w702:dbl, "LSI-D out[6]"=w701:dbl, "LSI-D out[7]"=w700:dbl)  [unwired: 1 out]
        n174 = local read "ref LSI-D"() -> (w708:refnum<file>)
        n175 = local read "Cycle #"() -> (w711:i32)
        n176 = Format Into String(format string="%d,%s,%10.4f,%10.4f,%5.6f,%5.6f,%5.6f,%5.6f,%5.6f,%5.6f,%5.6f,%5.6f\\n", initial string=w708, w711, w712, w713, w718, w707, w706, w705, w704, w703, w702, w701, w700) -> ()  [unwired: 1 in, 2 out]
      }
    }
    n177 = stacked-sequence {
      tunnel: w239 -> [w344]
      tunnel: [w317] -> w233
      tunnel: w234 -> [w263]
      tunnel: [w256] -> w232
      tunnel: w222 -> [w250]
      frame #0 {
        n178 = local read "current time"() -> (w316:timestamp)
        n179 = local read "DAQ sample #"() -> (w249:i32)
        n180 = local read "Cycle #"() -> (w313:i32)
        n181 = To Double Precision Float(number=w316) -> (double precision float=w357:dbl)
        n182 = call "LV_UNIX.vi"("current time"=w316) -> ("date/time string"=w314:string, "UNIX time (s)"=w315:dbl)  [unwired: 9 in]
        n183 = case shown="True" TRUE {
          tunnel: w357 -> [_ w395]
          tunnel: w315 -> [_ w396]
          tunnel: w314 -> [_ w394]
          tunnel: w313 -> [_ w397]
          frame False {
          }
          frame True {
            w399 = "%d,%s,%10.4f,%10.4f,%5.6f,%5.6f,%5.6f,%5.6f,%5.6f,%5.6f,%5.6f,%9.6f,%9.6f,%9.6f,%9.6f,%9.6f,%9.6f,%9.6f,%9.9e\\n" ("format string")
            n184 = local read "DAQ RAW"() -> (w391:dbl[])
            n185 = local read "DAQ AIN CONV"() -> (w375:dbl[])
            n186 = local read "ref RAW"() -> (w392:refnum<file>)
            n187 = Index Array(array=w391) -> (element #1=w390:dbl, element #2=w389:dbl, element #3=w388:dbl, element #4=w387:dbl, element #5=w386:dbl, element #6=w385:dbl, element #7=w384:dbl, element #8=w383:dbl, element #9=w382:dbl, element #10=w381:dbl, element #11=w380:dbl, element #12=w379:dbl, element #13=w378:dbl, element #14=w376:dbl, element #15=w377:dbl)  [unwired: 15 in]
            n188 = local read "ref DAQ"() -> (w393:refnum<file>)
            n189 = Format Into String(format string=w399, initial string=w392, w397, w394, w396, w395, w390, w389, w388, w387, w386, w385, w384, w383, w382, w381, w380, w379, w378, w376, w377) -> (error out=w398:errorcluster)  [unwired: 1 in, 1 out]
            n190 = Index Array(array=w375) -> (element #1=w374:dbl, element #2=w373:dbl, element #3=w372:dbl, element #4=w371:dbl, element #5=w370:dbl, element #6=w369:dbl, element #7=w368:dbl, element #8=w367:dbl, element #9=w366:dbl, element #10=w365:dbl, element #11=w364:dbl, element #12=w363:dbl, element #13=w362:dbl, element #14=w361:dbl, element #15=w360:dbl)  [unwired: 15 in]
            n191 = Format Into String(format string=w399, initial string=w393, error in=w398, w397, w394, w396, w395, w374, w373, w372, w371, w370, w369, w368, w367, w366, w365, w364, w363, w362, w361, w360) -> ()  [unwired: 2 out]
          }
        }
        n192 = call <vilib>:"DAQmx Read (Analog 2D DBL NChan NSamp).vi"("task/channels in"=w250, "number of samples per channel"=w249, "timeout"=100.0, "error in"=errorcluster {"status"=FALSE, "code"=0, "source"=""}) -> ("task out"=w256:refnum<k21>, "data"=w295:dbl[][], "error out"=w252:errorcluster)  [unwired: 9 in]
        n193 = local write "error out (DAQ AIN)"(w252) -> ()
        n194 = Index Array(array=w295, index (col)=0 ("disabled index (col)")) -> (element=w277:dbl[])  [unwired: 1 in]
        n195 = Index Array(array=w295, index (row) #1=0 ("index (row)"), index (row) #2=1 ("index (row)"), index (row) #3=2 ("index (row)"), index (row) #4=3 ("index (row)"), index (row) #5=4 ("disabled index (col)"), index (row) #6=5 ("index (col)"), index (row) #7=6 ("disabled index (row)"), index (row) #8=7 ("disabled index (row)"), index (row) #9=8 ("disabled index (row)"), index (row) #10=9 ("index (row)"), index (row) #11=10 ("index (row)"), index (row) #12=11 ("index (row)"), index (row) #13=12 ("index (row)"), index (row) #14=13 ("index (row)")) -> (element #1=w326:dbl[], element #2=w331:dbl[], element #3=w334:dbl[], element #4=w328:dbl[], element #5=w327:dbl[], element #6=w325:dbl[], element #7=w321:dbl[], element #8=w320:dbl[], element #9=w319:dbl[], element #10=w297:dbl[], element #11=w296:dbl[], element #12=w280:dbl[], element #13=w272:dbl[], element #14=w271:dbl[])  [unwired: 14 in]
        n196 = Array Size(array=w277) -> (size(s)=w276:i32)
        n197 = Insert Into Array(array=w277, index=w276, new element=0.0 ("new element/subarray")) -> (→"DAQ RAW":dbl[])
        n198 = stacked-sequence {
          tunnel: [w440 _ _ _ _ _ _ _ _ _ _ _ _ _] -> w343
          tunnel: [_ w449 _ _ _ _ _ _ _ _ _ _ _ _] -> w341
          tunnel: [_ _ w456 _ _ _ _ _ _ _ _ _ _ _] -> w340
          tunnel: w331 -> [_ w446 _ _ _ _ _ _ _ _ _ _ _ _]
          tunnel: [_ _ _ w465 _ _ _ _ _ _ _ _ _ _] -> w337
          tunnel: [_ _ _ _ w474 _ _ _ _ _ _ _ _ _] -> w336
          tunnel: [_ _ _ _ _ w483 _ _ _ _ _ _ _ _] -> w335
          tunnel: w334 -> [_ _ w455 _ _ _ _ _ _ _ _ _ _ _]
          tunnel: [_ _ _ _ _ _ w491 _ _ _ _ _ _ _] -> w333
          tunnel: w328 -> [_ _ _ w464 _ _ _ _ _ _ _ _ _ _]
          tunnel: w327 -> [_ _ _ _ w473 _ _ _ _ _ _ _ _ _]
          tunnel: w326 -> [w437 _ _ _ _ _ _ _ _ _ _ _ _ _]
          tunnel: w325 -> [_ _ _ _ _ w482 _ _ _ _ _ _ _ _]
          tunnel: w321 -> [_ _ _ _ _ _ w492 _ _ _ _ _ _ _]
          tunnel: w320 -> [_ _ _ _ _ _ _ w501 _ _ _ _ _ _]
          tunnel: w319 -> [_ _ _ _ _ _ _ _ w509 _ _ _ _ _]
          tunnel: [_ _ _ _ _ _ _ w500 _ _ _ _ _ _] -> w318
          tunnel: w297 -> [_ _ _ _ _ _ _ _ _ w520 _ _ _ _]
          tunnel: w296 -> [_ _ _ _ _ _ _ _ _ _ w531 _ _ _]
          tunnel: [_ _ _ _ _ _ _ _ _ w521 _ _ _ _] -> w286
          tunnel: [_ _ _ _ _ _ _ _ _ w519 _ _ _ _] -> _
          tunnel: [_ _ _ _ _ _ _ _ w510 _ _ _ _ _] -> w285
          tunnel: w280 -> [_ _ _ _ _ _ _ _ _ _ _ w537 _ _]
          tunnel: w272 -> [_ _ _ _ _ _ _ _ _ _ _ _ w546 _]
          tunnel: w271 -> [_ _ _ _ _ _ _ _ _ _ _ _ _ w550]
          tunnel: [_ _ _ _ _ _ _ _ _ _ _ _ _ w549] -> w269
          tunnel: [_ _ _ _ _ _ _ _ _ _ _ _ w540 _] -> w270
          tunnel: w249 -> [w436 w445 w454 w463 w472 w481 w490 w499 w508 w517 w530 w536 w539 w548]
          tunnel: [_ _ _ _ _ _ _ _ _ _ _ w534 _ _] -> w251
          tunnel: [_ _ _ _ _ _ _ _ _ _ w527 _ _ _] -> w248
          frame #0 {
            # "0"
            # "P (4K)"
            n199 = Add Array Elements(numeric array=w437) -> (sum=w439:dbl)
            n200 = Divide(x=w439, y=w436) -> (x/y=w438:dbl)
            n201 = call "scaling_calculator.vi"("x1"=1.0, "y1"=0.0 ("x1"), "x"=w438, "x2"=3.0 ("x1"), "y2"=100000.0 ("x1")) -> ("y"=w440:dbl)  [unwired: 2 in]
          }
          frame #1 {
            # "1"
            # "LM"
            n202 = Add Array Elements(numeric array=w446) -> (sum=w448:dbl)
            n203 = Divide(x=w448, y=w445) -> (x/y=w447:dbl)
            n204 = call "scaling_calculator.vi"("x1"=0.0, "y1"=0.0 ("x1"), "x"=w447, "x2"=0.1 ("x1"), "y2"=100.0 ("x1")) -> ("y"=w449:dbl)  [unwired: 2 in]
          }
          frame #2 {
            # "2"
            # "Delta P He3"
            n205 = Add Array Elements(numeric array=w455) -> (sum=w458:dbl)
            n206 = Divide(x=w458, y=w454) -> (x/y=w457:dbl)
            n207 = call "scaling_calculator.vi"("x1"=1.0, "y1"=0.0 ("x1"), "x"=w457, "x2"=5.0 ("x1"), "y2"=20000.0 ("x1")) -> ("y"=w456:dbl)  [unwired: 2 in]
          }
          frame #3 {
            # "3"
            # "Delta P He 4"
            n208 = Add Array Elements(numeric array=w464) -> (sum=w467:dbl)
            n209 = Divide(x=w467, y=w463) -> (x/y=w466:dbl)
            n210 = call "scaling_calculator.vi"("x1"=1.0, "y1"=0.0 ("x1"), "x"=w466, "x2"=5.0 ("x1"), "y2"=1000.0 ("x1")) -> ("y"=w465:dbl)  [unwired: 2 in]
          }
          frame #4 {
            # "4"
            # "FM He4"
            n211 = Add Array Elements(numeric array=w473) -> (sum=w476:dbl)
            n212 = Divide(x=w476, y=w472) -> (x/y=w475:dbl)
            n213 = call "scaling_calculator.vi"("x1"=0.0, "y1"=0.0 ("x1"), "x"=w475, "x2"=5.0 ("x1"), "y2"=500.0 ("x1")) -> ("y"=w474:dbl)  [unwired: 2 in]
          }
          frame #5 {
            # "5"
            # "FM He3"
            n214 = Add Array Elements(numeric array=w482) -> (sum=w485:dbl)
            n215 = Divide(x=w485, y=w481) -> (x/y=w484:dbl)
            n216 = call "scaling_calculator.vi"("x1"=0.0, "y1"=0.0 ("x1"), "x"=w484, "x2"=5.0 ("x1"), "y2"=200.0 ("x1")) -> ("y"=w483:dbl)  [unwired: 2 in]
          }
          frame #6 {
            # "LM1300"
            # "6"
            n217 = Add Array Elements(numeric array=w492) -> (sum=w498:dbl)
            n218 = Divide(x=w498, y=w490) -> (x/y=w497:dbl)
            n219 = call "scaling_calculator.vi"("x1"=0.0, "y1"=0.0 ("x1"), "x"=w497, "x2"=10.0 ("x1"), "y2"=100.0 ("x1")) -> ("y"=w491:dbl)  [unwired: 2 in]
          }
          frame #7 {
            # "7"
            # "AI16 absolute pressure"
            n220 = Add Array Elements(numeric array=w501) -> (sum=w507:dbl)
            n221 = Divide(x=w507, y=w499) -> (x/y=w502:dbl)
            n222 = call "scaling_calculator.vi"("x1"=1.0, "y1"=0.0 ("x1"), "x"=w502, "x2"=5.0 ("x1"), "y2"=200000.0 ("x1")) -> ("y"=w500:dbl)  [unwired: 2 in]
          }
          frame #8 {
            # "8"
            # "AI17 absolute pressure"
            n223 = Add Array Elements(numeric array=w509) -> (sum=w516:dbl)
            n224 = Divide(x=w516, y=w508) -> (x/y=w511:dbl)
            n225 = call "scaling_calculator.vi"("x1"=1.0, "y1"=0.0 ("x1"), "x"=w511, "x2"=5.0 ("x1"), "y2"=200000.0 ("x1")) -> ("y"=w510:dbl)  [unwired: 2 in]
          }
          frame #9 {
            # "9"
            # "AIN18 baratron front"
            n226 = Add Array Elements(numeric array=w520) -> (sum=w522:dbl)
            n227 = Divide(x=w522, y=w517) -> (x/y=w519:dbl)
            n228 = case shown="False" TRUE {
              tunnel: [w524 w525] -> w521
              tunnel: w519 -> [w523 w526]
              frame False {
                n229 = call "scaling_calculator_baratron.vi"("x"=w523) -> ("y (Pa)"=w524:dbl)  [unwired: 5 in, 1 out]
              }
              frame True {
                n230 = call "baratron_conv_analog.vi"("V_ana (V)"=w526) -> ("y (Pa)"=w525:dbl)  [unwired: 10 in]
              }
            }
          }
          frame #10 {
            # "10"
            # "AIN 19 baratron buffer 1\n--> in this version, changed to voltage readout of the heater"
            n231 = Add Array Elements(numeric array=w531) -> (sum=w532:dbl)
            n232 = Divide(x=w532, y=w530) -> (x/y=w529:dbl)
            n233 = Divide(x=w529, y="Rv/(Rv+Ro)") -> (x/y=w527:dbl)
          }
          frame #11 {
            # "11"
            # "AIN20 baratron buffer 2\n-->AIN23  Volage over 10Ohm resistor is converted to current"
            n234 = Add Array Elements(numeric array=w537) -> (sum=w538:dbl)
            n235 = Divide(x=w538, y=w536) -> (x/y=w535:dbl)
            n236 = Divide(x=w535, y="Ri (Ohm)") -> (x/y=w534:dbl)
          }
          frame #12 {
            # "AIN21 leak detector exp"
            n237 = Add Array Elements(numeric array=w546) -> (sum=w547:dbl)
            n238 = Divide(x=w547, y=w539) -> (x/y=w545:dbl)
            n239 = Round To Nearest(number=w545) -> (nearest integer value=w544:dbl)
            n240 = Add(x=w544, y=2.0) -> (x+y=w542:dbl)
            n241 = Multiply(x=w542, y=-1.0) -> (x*y=w540:dbl)
          }
          frame #13 {
            # "AIN21 leak detector mantissa"
            n242 = Add Array Elements(numeric array=w550) -> (sum=w551:dbl)
            n243 = Divide(x=w551, y=w548) -> (x/y=w549:dbl)
          }
        }
        n244 = Power Of 10(x=w270) -> (10^x=w268:dbl)
        n245 = Multiply(x=w269, y=w268) -> (x*y=w267:dbl)
        n246 = Build Array(w343, w341, w340, w337, w336, w335, w333, w318, w285, w286, w248, w251, w270, w269, w267) -> (w254:dbl[])
        "DAQ AIN CONV" <- w254
        n247 = local write "OUT S.1 1"(w254) -> ()
        n248 = local write "OUT S.1.2"(w254) -> ()
        n249 = Build Array (concatenate)(w344, w254) -> (w317:dbl[][])
        n250 = Index Array(array=w317, index (col) #1=0 ("disabled index (col)"), index (col) #2=1 ("disabled index (col)"), index (col) #3=2 ("disabled index (col)"), index (col) #4=3 ("disabled index (col)"), index (col) #5=4 ("index (col)"), index (col) #6=5 ("index (col)"), index (col) #7=6 ("index (col)"), index (col) #8=7 ("index (col)"), index (col) #9=8 ("index (col)"), index (col) #10=9 ("index (col)"), index (col) #11=10 ("index (col)"), index (col) #12=11 ("index (col)"), index (col) #13=12 ("index (col)"), index (col) #14=13 ("index (col)"), index (col) #15=14 ("index (col)")) -> (element #1=w355:dbl[], element #2=w353:dbl[], element #3=w351:dbl[], element #4=w349:dbl[], element #5=w346:dbl[], element #6=w345:dbl[], element #7=w279:dbl[], element #8=w278:dbl[], element #9=w308:dbl[], element #10=w291:dbl[], element #11=w289:dbl[], element #12=w283:dbl[], element #13=w262:dbl[], element #14=w261:dbl[], element #15=w260:dbl[])  [unwired: 15 in]
        n251 = Bundle(w263, w355) -> (w312:cluster{dbl[], dbl[]})  [unwired: 1 in]
        n252 = Bundle(w263, w353) -> (w311:cluster{dbl[], dbl[]})  [unwired: 1 in]
        n253 = Bundle(w263, w351) -> (w307:cluster{dbl[], dbl[]})  [unwired: 1 in]
        n254 = Bundle(w263, w349) -> (w306:cluster{dbl[], dbl[]})  [unwired: 1 in]
        n255 = Bundle(w263, w346) -> (w305:cluster{dbl[], dbl[]})  [unwired: 1 in]
        n256 = Bundle(w263, w345) -> (w304:cluster{dbl[], dbl[]})  [unwired: 1 in]
        n257 = Bundle(w263, w279) -> (w303:cluster{dbl[], dbl[]})  [unwired: 1 in]
        n258 = Bundle(w263, w278) -> (w302:cluster{dbl[], dbl[]})  [unwired: 1 in]
        n259 = Bundle(w263, w308) -> (w301:cluster{dbl[], dbl[]})  [unwired: 1 in]
        n260 = Bundle(w263, w291) -> (w290:cluster{dbl[], dbl[]})  [unwired: 1 in]
        n261 = Bundle(w263, w289) -> (w288:cluster{dbl[], dbl[]})  [unwired: 1 in]
        n262 = Bundle(w263, w283) -> (w282:cluster{dbl[], dbl[]})  [unwired: 1 in]
        n263 = Bundle(w263, w262) -> (w259:cluster{dbl[], dbl[]})  [unwired: 1 in]
        n264 = Bundle(w263, w261) -> (w258:cluster{dbl[], dbl[]})  [unwired: 1 in]
        n265 = Bundle(w263, w260) -> (w257:cluster{dbl[], dbl[]})  [unwired: 1 in]
        n266 = Build Array(w312, w311, w307, w306, w305, w304, w303, w302, w301, w290, w288, w282, w259, w258, w257) -> (w300:cluster{dbl[], dbl[]}[])
        n267 = stacked-sequence {
          tunnel: w300 -> [w405 w417 w429]
          frame #0 {
            n268 = local read "DAQ AIN CH indic."() -> (w402:string[])
            n269 = Array Size(array=w402) -> (size(s)=w404:i32)
            n270 = for {
              N: w404 -> [_]
              tunnel: [w409] -> w403
              tunnel: w402 -> [w408] mode=indexing
              i -> [w411]
              n271 = control-ref of="Graph S.1.1"() -> (w407:refnum<vi>)
              n272 = property class="XYGraph (strict)"(reference=w407, error in=errorcluster {"status"=FALSE, "code"=0, "source"=""} ("error in (no error)"), "Active Plot"=w411, "Plot.Plot Name"=w408) -> (error out=w409:errorcluster)  [unwired: 1 out]
            }
            n273 = control-ref of="Graph S.1.1"() -> (w401:refnum<vi>)
            n274 = property class="XYGraph (strict)"(reference=w401, error in=w403, "Val(Sgnl)"=w405) -> (error out=w406:errorcluster)  [unwired: 1 out]
            n275 = control-ref of="error out (decoration)"() -> (w400:refnum<vi>)
            n276 = property class="Clust (strict)"(reference=w400, "Value"=w406) -> ()  [unwired: 1 in, 2 out]
          }
          frame #1 {
            n277 = local read "DAQ AIN CH indic."() -> (w414:string[])
            n278 = Array Size(array=w414) -> (size(s)=w416:i32)
            n279 = for {
              N: w416 -> [_]
              tunnel: [w421] -> w415
              tunnel: w414 -> [w420] mode=indexing
              i -> [w423]
              n280 = control-ref of="Graph S.1.2"() -> (w419:refnum<vi>)
              n281 = property class="XYGraph (strict)"(reference=w419, error in=errorcluster {"status"=FALSE, "code"=0, "source"=""} ("error in (no error)"), "Active Plot"=w423, "Plot.Plot Name"=w420) -> (error out=w421:errorcluster)  [unwired: 1 out]
            }
            n282 = control-ref of="Graph S.1.2"() -> (w412:refnum<vi>)
            n283 = property class="XYGraph (strict)"(reference=w412, error in=w415, "Val(Sgnl)"=w417) -> (error out=w418:errorcluster)  [unwired: 1 out]
            n284 = control-ref of="error out (decoration)"() -> (w413:refnum<vi>)
            n285 = property class="Clust (strict)"(reference=w413, "Value"=w418) -> ()  [unwired: 1 in, 2 out]
          }
          frame #2 {
            n286 = local read "DAQ AIN CH indic."() -> (w426:string[])
            n287 = control-ref of="Graph S.1.3"() -> (w424:refnum<vi>)
            n288 = Array Size(array=w426) -> (size(s)=w428:i32)
            n289 = for {
              N: w428 -> [_]
              tunnel: [w433] -> w427
              tunnel: w426 -> [w432] mode=indexing
              tunnel: w424 -> [w431]
              i -> [w435]
              n290 = property class="XYGraph (strict)"(reference=w431, error in=errorcluster {"status"=FALSE, "code"=0, "source"=""} ("error in (no error)"), "Active Plot"=w435, "Plot.Plot Name"=w432) -> (error out=w433:errorcluster)  [unwired: 1 out]
            }
            n291 = property class="XYGraph (strict)"(reference=w424, error in=w427, "Val(Sgnl)"=w429) -> (error out=w430:errorcluster)  [unwired: 1 out]
            n292 = control-ref of="error out (decoration)"() -> (w425:refnum<vi>)
            n293 = property class="Clust (strict)"(reference=w425, "Value"=w430) -> ()  [unwired: 1 in, 2 out]
          }
        }
      }
    }
    n294 = local read "DAQ AOUT task out"() -> (w224:refnum<k21>)
    "Cycle #" <- w240
  }
  n295 = while {
    tunnel: w6 -> [w745]
    tunnel: [w745] -> w15
    shift-right: [w737] -> _
    shift-left: w9 -> [w739]
    shift-right: [w736] -> _
    shift-left: w9 -> [w738]
    i -> [w740]
    stop <- "stop" stop-if-true
    n296 = event shown="[0] \"DAQ OUT SET V\", \"DAQ OUT ON?\": Value Change" {
      selector: _ -> [_ _ _]
      dyn-events: _ -> [_ _ _]
      timeout: _ -> [_ _ _]
      tunnel: [w762 errorcluster {"status"=FALSE, "code"=0, "source"=""} ("error out") errorcluster {"status"=FALSE, "code"=0, "source"=""} ("error out")] -> w742
      tunnel: [_ TRUE _] -> _
      tunnel: w738 -> [w757 w785 w788]
      tunnel: [w755 w785 w788] -> w736
      tunnel: w739 -> [w754 w786 w789]
      tunnel: [w753 w786 w789] -> w737
      event "DAQ OUT SET V", "DAQ OUT ON?": Value Change {
        w747 = 11.0 ("y")
        # "return x only when 0<=x<=10"
        n297 = event-data() -> ()  [unwired: 1 in, 6 out]
        n298 = Get Date/Time In Seconds() -> (seconds since 1Jan1904=w752:timestamp)
        n299 = local read "V_lim_max"() -> (w750:dbl)
        n300 = local read "V_lim_min"() -> (w748:dbl)
        n301 = To Double Precision Float(number=w752) -> (double precision float=w751:dbl)
        n302 = Multiply(x=w748, y=w747) -> (x*y=w746:dbl)
        n303 = Multiply(x=w750, y=w747) -> (x*y=w749:dbl)
        n304 = Build Array (concatenate)(w754, w751) -> (w753:dbl[])
        n305 = Greater?(x="DAQ OUT SET V", y=w749) -> (0:w760:bool)
        n306 = case shown="False" w760 {
          tunnel: w746 -> [w766 _]
          tunnel: "DAQ OUT SET V" -> [w763 _]
          tunnel: [w764 w769] -> w759
          frame False {
            n307 = Less?(x=w763, y=w766) -> (x < y?=w765:bool)
            n308 = case shown="False" w765 {
              tunnel: [w767 w768] -> w764
              tunnel: w763 -> [w767 _]
              frame False {
              }
              frame True {
                w768 = 0.0 ("y")
                n309 = property on="DAQ OUT SET V" class="DigNum (strict)"("Val(Sgnl)"=w768) -> ()  [unwired: 2 in, 2 out]
              }
            }
          }
          frame True {
            w769 = 110.0 ("y")
            n310 = property on="DAQ OUT SET V" class="DigNum (strict)"("Val(Sgnl)"=w769) -> ()  [unwired: 2 in, 2 out]
          }
        }
        n311 = case shown="False" "DAQ OUT ON?" {
          tunnel: [w771 w782] -> w762
          tunnel: [w770 w777] -> w756
          tunnel: w759 -> [_ w777]
          frame False {
            w770 = 0.0 ("element")
            n312 = local read "DAQ AOUT task out"() -> (w775:refnum<k21>)
            n313 = Build Array(w770) -> (w772:dbl[])
            n314 = call <vilib>:"DAQmx Write (Analog 1D DBL 1Chan NSamp).vi"("task/channels in"=w775, "data"=w772, "timeout"=100.0) -> ("task out"=w774:refnum<k21>, "error out"=w771:errorcluster)  [unwired: 10 in, 1 out]
            n315 = local write "DAQ AOUT task out"(w774) -> ()
          }
          frame True {
            # "Vset = 110/10 * Vctrl\ntherefore \nVctrl = Vset / 11.0"
            n316 = Divide(x=w777, y=11.0) -> (x/y=w776:dbl)
            "Vctrl" <- w776
            n317 = local read "DAQ AOUT task out"() -> (w781:refnum<k21>)
            n318 = Build Array(w776) -> (w779:dbl[])
            n319 = call <vilib>:"DAQmx Write (Analog 1D DBL 1Chan NSamp).vi"("task/channels in"=w781, "data"=w779, "timeout"=100.0) -> ("task out"=w780:refnum<k21>, "error out"=w782:errorcluster)  [unwired: 10 in, 1 out]
            n320 = local write "DAQ AOUT task out"(w780) -> ()
          }
        }
        n321 = Build Array (concatenate)(w757, w756) -> (w755:dbl[])
      }
      event "stop": Value Change {
        n322 = event-data() -> ()  [unwired: 1 in, 6 out]
      }
      event Timeout {
        n323 = event-data() -> ()  [unwired: 1 in, 3 out]
      }
    }
    "error out (DAQ AOU)" <- w742
    n324 = Wait (ms)(milliseconds to wait=u32 50) -> ()  [unwired: 1 out]
    n325 = Bundle(w737, w736) -> (→"Graph V SET":cluster{dbl[], dbl[]})  [unwired: 1 in]
    "cycle # CTRL" <- w740
  }
  n326 = while {
    tunnel: w6 -> [w818]
    tunnel: [w817] -> w10
    tunnel: w5 -> [w804]
    shift-right: [w801] -> _
    shift-left: w5 -> [w793]
    shift-right: [w800] -> _
    shift-left: w5 -> [w799]
    shift-right: [w796] -> _
    shift-left: w5 -> [w795]
    i -> [w820]
    stop <- w819 stop-if-true
    n327 = Wait (ms)(milliseconds to wait="dt (ms) (>50)") -> ()  [unwired: 1 out]
    n328 = stacked-sequence {
      seq-local: [_ _ _ w874 _] -> [_ _ _ _ w882]
      seq-local: [_ _ _ w873 _] -> [_ _ _ _ w881]
      seq-local: [_ _ _ w871 _] -> [_ _ _ _ w880]
      tunnel: w793 -> [w824 _ _ _ _]
      tunnel: w799 -> [w825 _ _ _ _]
      tunnel: w795 -> [w826 _ _ _ _]
      tunnel: [_ _ _ _ w882] -> w803
      tunnel: [_ _ _ _ w881] -> w802
      tunnel: [_ _ _ _ w880] -> w794
      frame #0 {
        n329 = local write "Array dT"(w824) -> ()
        n330 = local write "Array Q"(w825) -> ()
        n331 = local write "Array time"(w826) -> ()
      }
      frame #1 {
        n332 = case shown="True" "Record Boling curve" {
          frame False {
          }
          frame True {
            # "Write the column names"
            n333 = Get Date/Time In Seconds() -> (seconds since 1Jan1904=w854:timestamp)
            n334 = Format Date/Time String(time format string (%c)="%Y%m%d_%H%M%S_", seconds (now)=w854) -> (date/time string=w856:string)  [unwired: 1 in]
            n335 = Concatenate Strings("BC_" ("string"), w856, "BC file comment") -> (w838:string)
            n336 = local read "base path"() -> (w839:path)
            n337 = local read "base path"() -> (w857:path)
            n338 = Concatenate Strings(w838, ".csv" ("string")) -> (w840:string)
            n339 = Concatenate Strings(w838, ".bmp" ("string")) -> (w836:string)
            n340 = Build Path(base path=w839, name or relative path=w836) -> (appended path=w835:path)
            n341 = Build Path(base path=w857, name or relative path=w840) -> (appended path=w858:path)
            n342 = invoke on="Graph BC" class="XYGraph (strict)" method="Export Image"("FileType"=enum32{"BMP", "EPS", "EMF", "PICT"}."BMP" ("File Type"), "Target"=enum32{"File", "Clipboard"}."File", "Path"=w835, "HideGrid"=FALSE ("Hide Grid"), "Overwrite"=TRUE ("Always Overwrite")) -> ()  [unwired: 3 in, 8 out]
            n343 = Open/Create/Replace File(file path (use dialog)=w858, error in=errorcluster {"status"=FALSE, "code"=0, "source"=""}, operation (0:open)=T2."create") -> (refnum out=w859:refnum<file>, error out=w860:errorcluster)  [unwired: 3 in, 1 out]
            n344 = local read "Array time"() -> (w830:dbl[])
            n345 = local read "Array dT"() -> (w828:dbl[])
            n346 = local read "Array Q"() -> (w829:dbl[])
            n347 = Format Into String(format string="%s,%s,%s,%s,%s\\n" ("time format string (%c)"), initial string=w859, error in=w860, "INDEX" ("input 1"), "Datetime" ("input 1"), "UNIX_time" ("input 1"), "Q (W)" ("input 4"), "dT (K)" ("input 5")) -> (resulting string=w842:refnum<file>)  [unwired: 1 out]
            n348 = Array Size(array=w830) -> (size(s)=w843:i32)
            n349 = for {
              N: w843 -> [_]
              tunnel: w842 -> [w869]
              tunnel: w830 -> [w867] mode=indexing
              tunnel: w829 -> [w862] mode=indexing
              tunnel: w828 -> [w861] mode=indexing
              i -> [w865]
              n350 = To Time Stamp(1:w867) -> (0:w866:timestamp)
              n351 = call "LV_UNIX.vi"("current time"=w866) -> ("date/time string"=w864:string, "UNIX time (s)"=w863:dbl)  [unwired: 9 in]
              n352 = Format Into String(format string="%d,%s,%10.9f,%10.9f,%10.9f\\n", initial string=w869, w865, w864, w863, w862, w861) -> ()  [unwired: 1 in, 2 out]
            }
          }
        }
      }
      frame #2 {
        n353 = local write "Record Boling curve"(FALSE ("Record Boling curve")) -> ()
      }
      frame #3 {
        n354 = case shown="False" "Refresh boiling curve" {
          tunnel: [w877 w878] -> w874
          tunnel: [w876 w878] -> w873
          tunnel: [w875 w878] -> w871
          frame False {
            n355 = local read "Array time"() -> (w875:dbl[])
            n356 = local read "Array dT"() -> (w877:dbl[])
            n357 = local read "Array Q"() -> (w876:dbl[])
          }
          frame True {
            w878 = dbl[] []
          }
        }
      }
      frame #4 {
        n358 = local write "Refresh boiling curve"(FALSE ("Boling curve \nRefresh")) -> ()
      }
    }
    n359 = flat-sequence {
      tunnel: w820 -> [_]
      frame #0 {
        n360 = case shown="True" "DAQ-O \nAUTO CTL" {
          frame False {
          }
          frame True {
            n361 = local read "DAQ OUT SET V"() -> (w884:dbl)
            n362 = local read "DAQ OUT MAX (V)"() -> (w888:dbl)
            n363 = local read "DAQ OUT MIN (V)"() -> (w887:dbl)
            n364 = Add(x="dV/cycle (V)", y=w884) -> (x+y=w885:dbl)
            n365 = In Range and Coerce(upper limit=w888, x=w885, lower limit=w887) -> (In Range?=w886:bool)  [unwired: 1 out]
            n366 = case shown="True" w886 {
              tunnel: w884 -> [_ _]
              tunnel: w885 -> [_ w891]
              tunnel: w884 -> [w890 _]
              frame False {
                n367 = property on="DAQ OUT SET V" class="DigNum (strict)"("Val(Sgnl)"=w890) -> ()  [unwired: 2 in, 2 out]
              }
              frame True {
                n368 = property on="DAQ OUT SET V" class="DigNum (strict)"("Val(Sgnl)"=w891) -> ()  [unwired: 2 in, 2 out]
              }
            }
          }
        }
      }
    }
    n369 = property on="stop" class="Bool (strict)"(error in=w818) -> (error out=w817:errorcluster, "Value"=w819:bool)  [unwired: 1 in, 1 out]
    n370 = local read "OUT S.1 1"() -> (w812:dbl[])
    n371 = case shown="False" "Select LSI 218/336" {
      tunnel: [w822 w823] -> w816
      frame False {
        n372 = local read "LSI-U out"() -> (w822:dbl[])
      }
      frame True {
        n373 = local read "LSI-D out"() -> (w823:dbl[])
      }
    }
    n374 = Index Array(array=w812, index=10) -> (element=w807:dbl)
    "V (V)" <- w807
    n375 = Index Array(array=w812, index=11) -> (element=w806:dbl)
    "I (A)" <- w806
    n376 = Index Array(array=w816, index=1) -> (element=w810:dbl)
    "T_Cu (K)" <- w810
    n377 = Index Array(array=w816, index=0) -> (element=w809:dbl)
    "T_He (K)" <- w809
    n378 = Get Date/Time In Seconds() -> (seconds since 1Jan1904=w798:timestamp)
    n379 = Subtract(x=w810, y=w809) -> (x-y=w808:dbl)
    n380 = Multiply(x=w807, y=w806) -> (x*y=w792:dbl)
    "P (W)" <- w792
    n381 = To Double Precision Float(number=w798) -> (double precision float=w797:dbl)
    n382 = Build Array (concatenate)(w803, w808) -> (w801:dbl[])
    n383 = Build Array (concatenate)(w794, w797) -> (w796:dbl[])
    n384 = Build Array (concatenate)(w802, w792) -> (w800:dbl[])
    n385 = Bundle(w801, w800) -> (→"Graph BC":cluster{dbl[], dbl[]})  [unwired: 1 in]
    "Array dT" <- w804
    "Array Q" <- w804
    "Array time" <- w804
  }
  n386 = Merge Errors(w16, w15, w14, w10) -> (w17:errorcluster)
  n387 = call <vilib>:"DAQmx Stop Task.vi"("task/channels in"=w24, "error in"=w17) -> ("task out"=w26:refnum<k21>, "error out"=w25:errorcluster)  [unwired: 12 in]
  n388 = call <vilib>:"DAQmx Clear Task.vi"("task in"=w26, "error in"=w25) -> ("error out"=w28:errorcluster)  [unwired: 13 in]
  n389 = call <vilib>:"DAQmx Stop Task.vi"("task/channels in"=w23, "error in"=w28) -> ("task out"=w29:refnum<k21>, "error out"=w27:errorcluster)  [unwired: 12 in]
  n390 = call <vilib>:"DAQmx Clear Task.vi"("task in"=w29, "error in"=w27) -> ("error out"=w8:errorcluster)  [unwired: 13 in]
  n391 = invoke on="stop" class="Bool (strict)" method="Reinit To Default"(error in=w8) -> (error out=→"error out (end)":errorcluster)  [unwired: 2 in, 2 out]
